vi "Parameter.vi"(9 "In":string, 10 "VIId":string, 11 "VariablesRef":T3) -> ()   [LabVIEW 2018, in "Array.lvlib"]
uses:
  Array.lvlib
  <userlib>/_OpenG.lib/dictionary/dictionary.llb/Dictionary Object RefNum__ogtk.ctl
  <userlib>/_OpenG.lib/dictionary/dictionary.llb/Dictionary Object RefNum - Enum__ogtk.ctl
  <vilib>/addons/_JKI.lib/Serialization/JSON/JKI JSON Serialization.lvlib
panel:
  in  "Tab Control":enum32{"Config", "控件"}(tab)
  in  "ArrayType":T1(tab)
  in  "索引_ArrayIndex":u32 caption="索引"
  in  "第一个元素_BuildArray":string(combo) caption="第一个元素"
  in  "第二个元素_BuildArray":string(combo) caption="第二个元素"
  in  "索引_InsertIntoArray":u32 caption="索引"
  in  "子数组_InsertIntoArray":string(combo) caption="子数组"
  in  "索引_DeleteFromArray":u32 caption="索引"
  in  "删除长度_DeleteFromArray":u32 caption="删除长度"
  in  "尺寸_InitializeArray":u32 caption="尺寸"
  in  "元素_InitializeArray":string(combo) caption="元素"
  in  "长度_ArraySubset":u32 caption="长度"
  in  "索引_ArraySubset":u32 caption="索引"
  in  "元素_SearchArray":string(combo) caption="元素"
  in  "起始索引_SearchArray":u32 caption="起始索引"
  in  "子数组_ReplaceArraySubset":string(combo) caption="子数组"
  in  "索引_ReplaceArraySubset":u32 caption="索引"
  in  "忽略NaN_ArrayAverage":bool
  in  "分隔符_ArrayToString":string(combo) caption="分隔符"
  in  "数组变量(ArrayVar)":u16(ring) items=["", "SN", "FileName", "ProductName", "TestLine", "TestStation"]
  in  "方法(Method)":T2(ring)
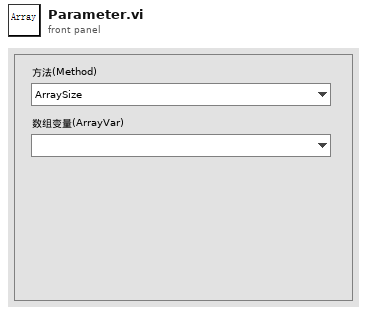
[diagram p1: front panel]
types:
  T1 = enum32{"ArraySize", "ArrayIndex", "BuildArray", "InsertIntoArray", "DeleteFromArray", "InitializeArray", "ArraySubset", "ArrayMax", "ArrayMin", "SearchArray", "ReplaceArraySubset", "SortArray", "ReverseArray", "ArrayAverage", "RemoveDuplicatesFromArray", "ArrayToString"}
  T2 = enum16{"ArraySize", "IndexArray", "BuildArray", "InsertIntoArray", "DeleteFromArray", "InitializeArray", "ArraySubset", "ArrayMax", "ArrayMin", "SearchArray", "ReplaceArraySubset", "SortArray", "ReverseArray", "ArrayAverage", "RemoveDuplicatesFromArray", "ArrayToString"}
  T3 = typedef "Dictionary Object RefNum__ogtk.ctl" = refnum<k1>
  T4 = cluster{"ArraySize":cluster{"json":cluster{"Method":string, "ArrayVar":string}}, "IndexArray":cluster{"json":cluster{"Method":string, "ArrayVar":string, "Index":i32}}, "BuildArray":cluster{"json":cluster{"Method":string, "FirstElementVar":string, "SecondElementVar":string}}, "InsertIntoArray":cluster{"json":cluster{"Method":string, "ArrayVar":string, "Index":i32, "SubArrayVar":string}}, "DeleteFromArray":cluster{"json":cluster{"Method":string, "ArrayVar":string, "Index":i32, "Length":i32}}, "InitializeArray":cluster{"json":cluster{"Method":string, "ElementVar":string, "DimensionSize":i32}}, "ArraySubset":cluster{"json":cluster{"Method":string, "ArrayVar":string, "Index":i32, "Length":i32}}, "ArrayMax":cluster{"json":cluster{"Method":string, "ArrayVar":string}}, "ArrayMin":cluster{"json":cluster{"Method":string, "ArrayVar":string}}, "SearchArray":cluster{"json":cluster{"Method":string, "ArrayVar":string, "ElementVar":string, "StartIndex":i32}}, "ReplaceArraySubset":cluster{"json":cluster{"Method":string, "ArrayVar":string, "Index":i32, "SubArrayVar":string}}, "SortArray":cluster{"json":cluster{"Method":string, "ArrayVar":string}}, "ReverseArray":cluster{"json":cluster{"Method":string, "ArrayVar":string}}, "ArrayAverage":cluster{"json":cluster{"Method":string, "NumArrayVar":string, "IgnoreNaN":bool}}, "RemoveDuplicatesFromArray":cluster{"json":cluster{"Method":string, "ArrayVar":string}}, "ArrayToString":cluster{"json":cluster{"Method":string, "ArrayVar":string, "Delimiter":string}}}
  T5 = enum32{"Invalid", "Standard", "Closed", "Hidden", "Minimized", "Maximized"}
  T6 = enum32{"invalid app kind", "Development System", "Run Time System", "Student Edition", "Embedded LabVIEW", "Evaluation", "Custom"}
  T7 = cluster{"Core":cluster{"Current VI Reference":refnum<vi>, "Close Panel on Exit?":bool}, "Parameter":cluster{"VariableRef":T3}, "Synchronize":cluster{"EnqueueData":cluster{"Action":enum16{"Create", "Query", "Revert", "UpdateVariable", "Close"}, "Data":variant}, "Echo":cluster{"VIRef":refnum<vi>, "JsonOut":string, "Status":string}, "Communicate":cluster{"ID":string, "JsonIn":string, "VarRef":T3}, "Queue":refnum<queue>}, "ArrayClusters":cluster{"ArraySize":cluster{"json":cluster{"Method":string, "ArrayVar":string}}, "IndexArray":cluster{"json":cluster{"Method":string, "ArrayVar":string, "Index":i32}}, "BuildArray":cluster{"json":cluster{"Method":string, "FirstElementVar":string, "SecondElementVar":string}}, "InsertIntoArray":cluster{"json":cluster{"Method":string, "ArrayVar":string, "Index":i32, "SubArrayVar":string}}, "DeleteFromArray":cluster{"json":cluster{"Method":string, "ArrayVar":string, "Index":i32, "Length":i32}}, "InitializeArray":cluster{"json":cluster{"Method":string, "ElementVar":string, "DimensionSize":i32}}, "ArraySubset":cluster{"json":cluster{"Method":string, "ArrayVar":string, "Index":i32, "Length":i32}}, "ArrayMax":cluster{"json":cluster{"Method":string, "ArrayVar":string}}, "ArrayMin":cluster{"json":cluster{"Method":string, "ArrayVar":string}}, "SearchArray":cluster{"json":cluster{"Method":string, "ArrayVar":string, "ElementVar":string, "StartIndex":i32}}, "ReplaceArraySubset":cluster{"json":cluster{"Method":string, "ArrayVar":string, "Index":i32, "SubArrayVar":string}}, "SortArray":cluster{"json":cluster{"Method":string, "ArrayVar":string}}, "ReverseArray":cluster{"json":cluster{"Method":string, "ArrayVar":string}}, "ArrayAverage":cluster{"json":cluster{"Method":string, "NumArrayVar":string, "IgnoreNaN":bool}}, "RemoveDuplicatesFromArray":cluster{"json":cluster{"Method":string, "ArrayVar":string}}, "ArrayToString":cluster{"json":cluster{"Method":string, "ArrayVar":string, "Delimiter":string}}}}
  T8 = cluster{"EnqueueData":cluster{"Action":enum16{"Create", "Query", "Revert", "UpdateVariable", "Close"}, "Data":variant}, "Echo":cluster{"VIRef":refnum<vi>, "JsonOut":string, "Status":string}, "Communicate":cluster{"ID":string, "JsonIn":string, "VarRef":T3}, "Queue":refnum<queue>}
  T9 = cluster{"Current VI Reference":refnum<vi>, "Close Panel on Exit?":bool}
  T10 = cluster{"json":cluster{"Method":string, "ArrayVar":string}}
  T11 = cluster{"json":cluster{"Method":string, "ArrayVar":string, "Index":i32}}
  T12 = cluster{"json":cluster{"Method":string, "FirstElementVar":string, "SecondElementVar":string}}
  T13 = cluster{"json":cluster{"Method":string, "ArrayVar":string, "Index":i32, "SubArrayVar":string}}
  T14 = cluster{"json":cluster{"Method":string, "ArrayVar":string, "Index":i32, "Length":i32}}
  T15 = cluster{"json":cluster{"Method":string, "ElementVar":string, "DimensionSize":i32}}
  T16 = cluster{"json":cluster{"Method":string, "ArrayVar":string, "ElementVar":string, "StartIndex":i32}}
  T17 = cluster{"json":cluster{"Method":string, "NumArrayVar":string, "IgnoreNaN":bool}}
  T18 = cluster{"json":cluster{"Method":string, "ArrayVar":string, "Delimiter":string}}
  T19 = cluster{"Action":enum16{"Create", "Query", "Revert", "UpdateVariable", "Close"}, "Data":variant}
  T20 = cluster{"ID":string, "JsonIn":string, "VarRef":T3}
  T21 = enum16{"Create", "Query", "Revert", "UpdateVariable", "Close"}
  T22 = cluster{"VIRef":refnum<vi>, "JsonOut":string, "Status":string}
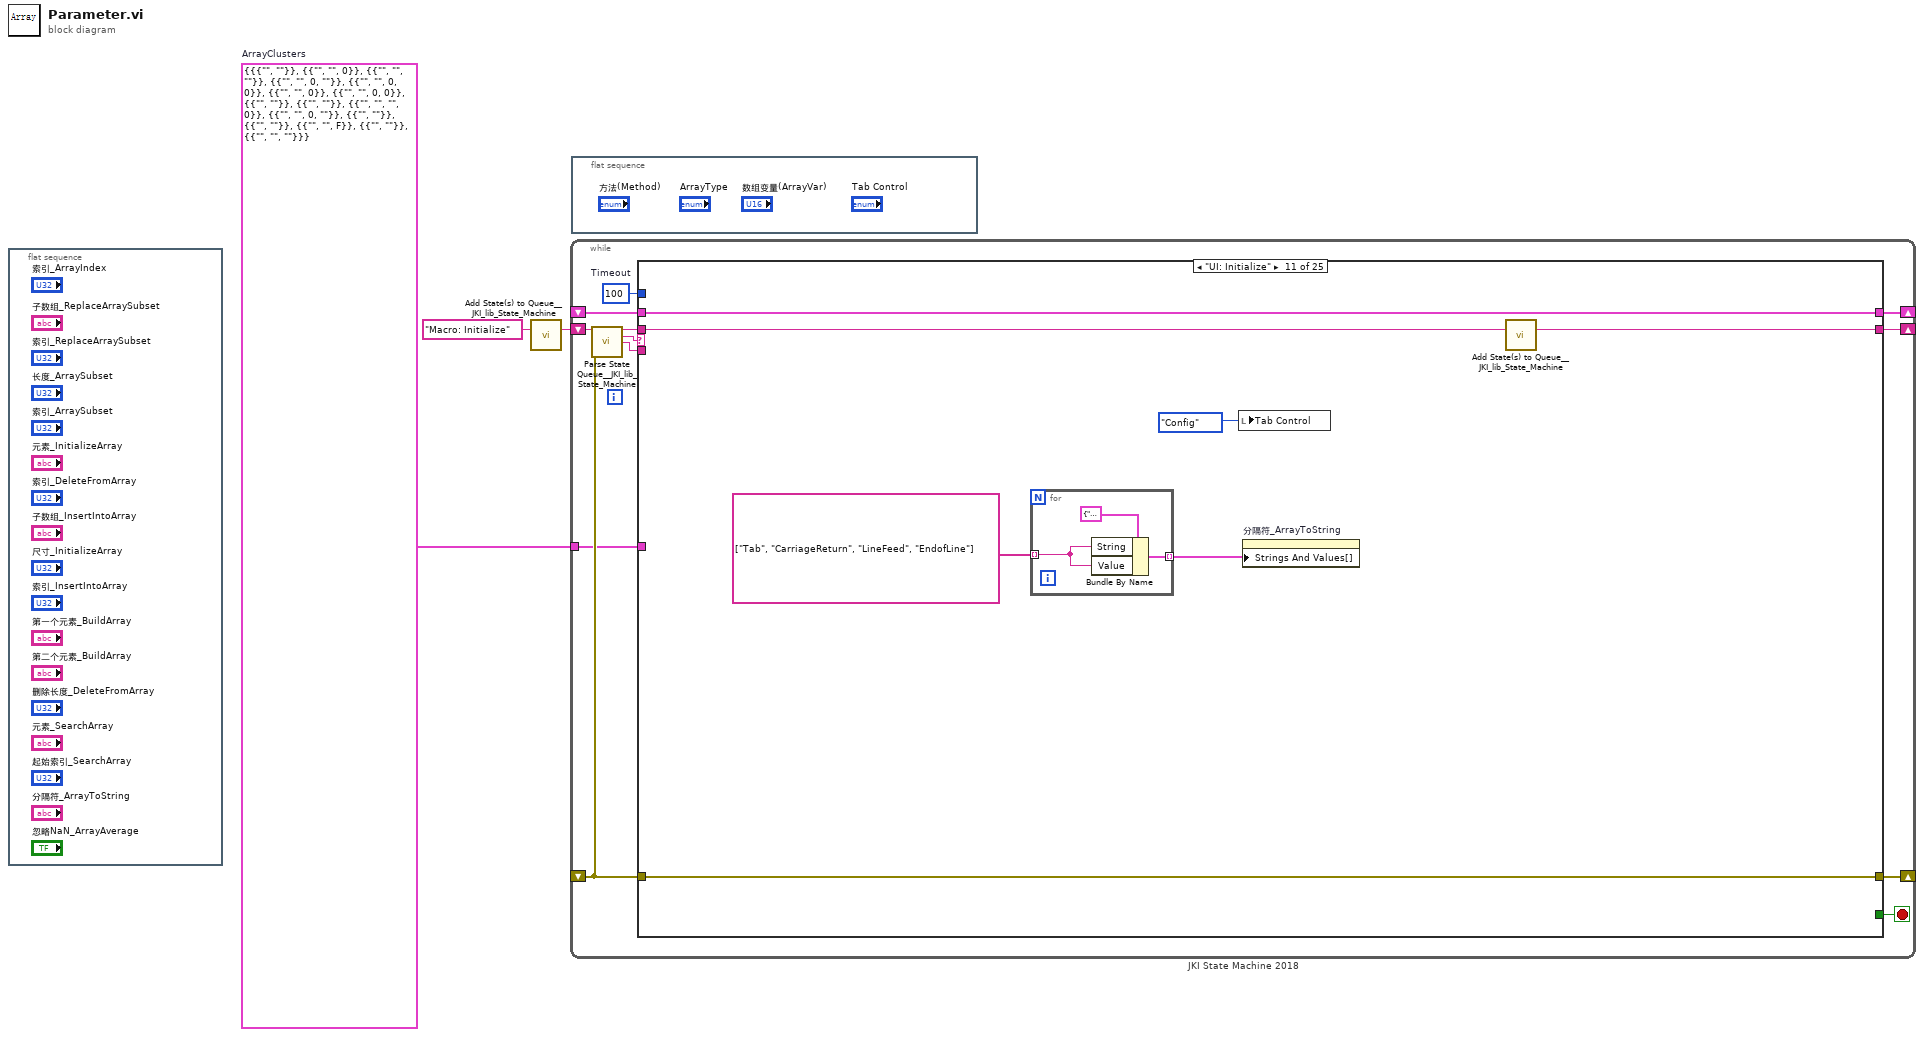
[diagram p0: block diagram]
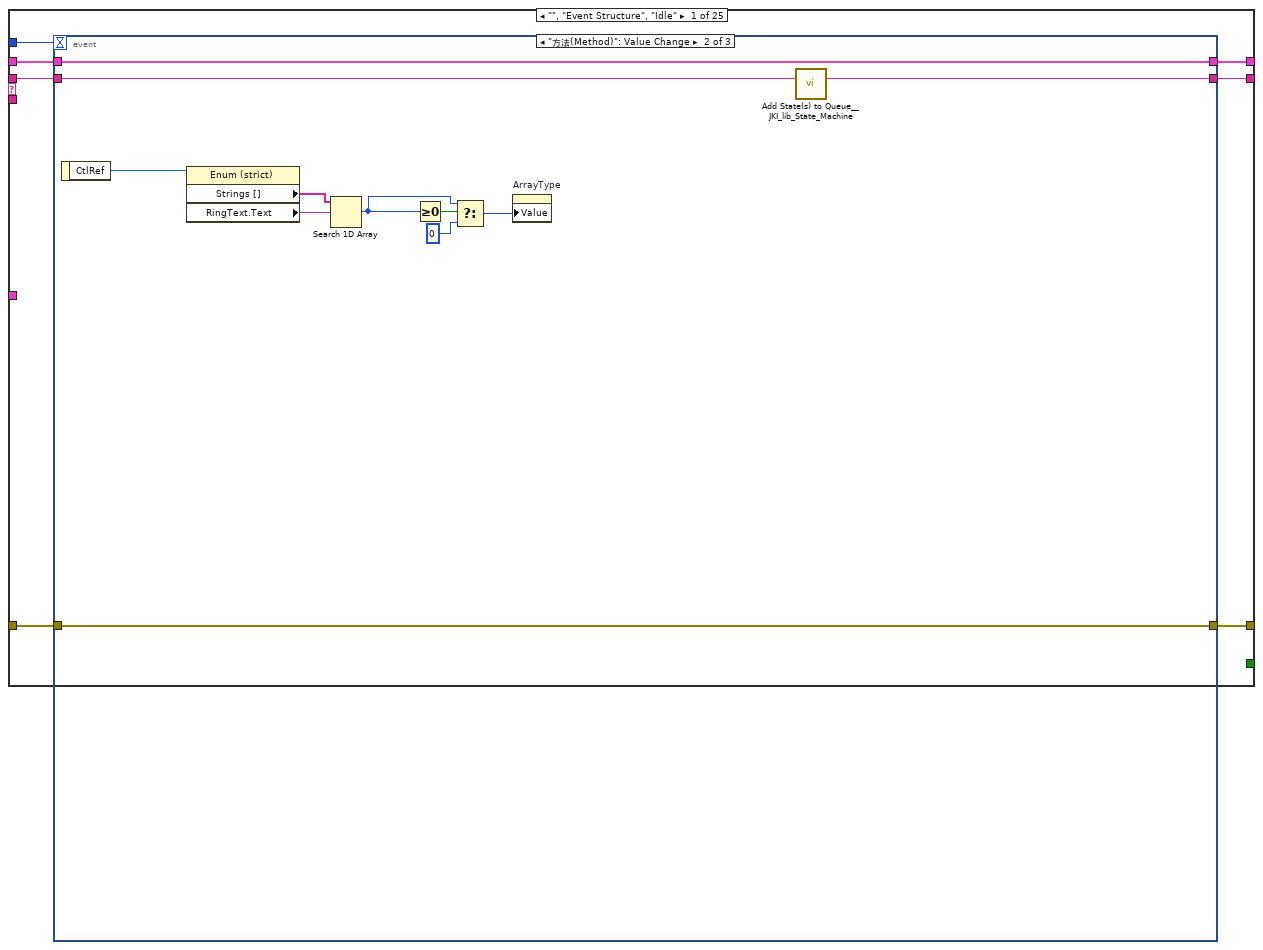
[diagram p2: hidden frame]
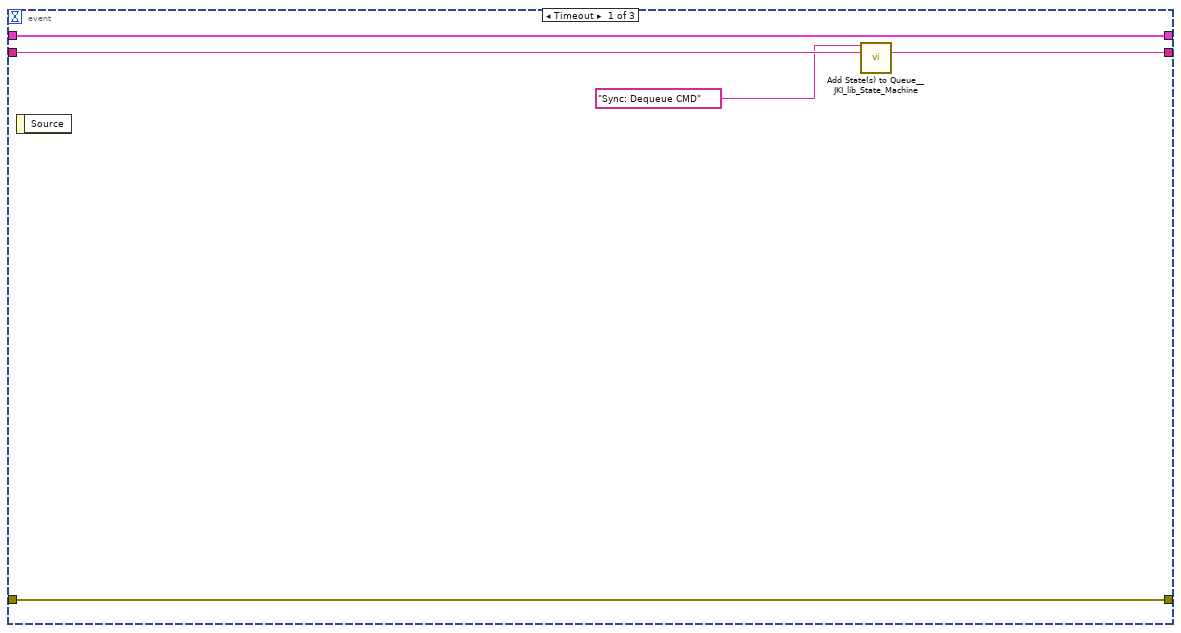
[diagram p3: hidden frame]
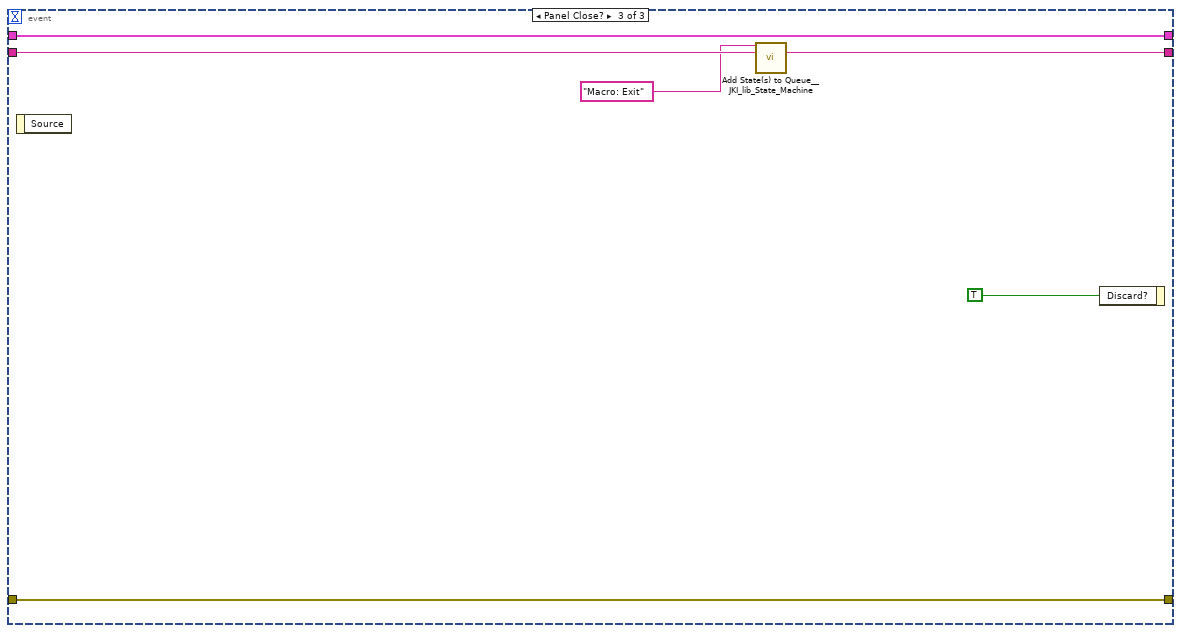
[diagram p4: hidden frame]
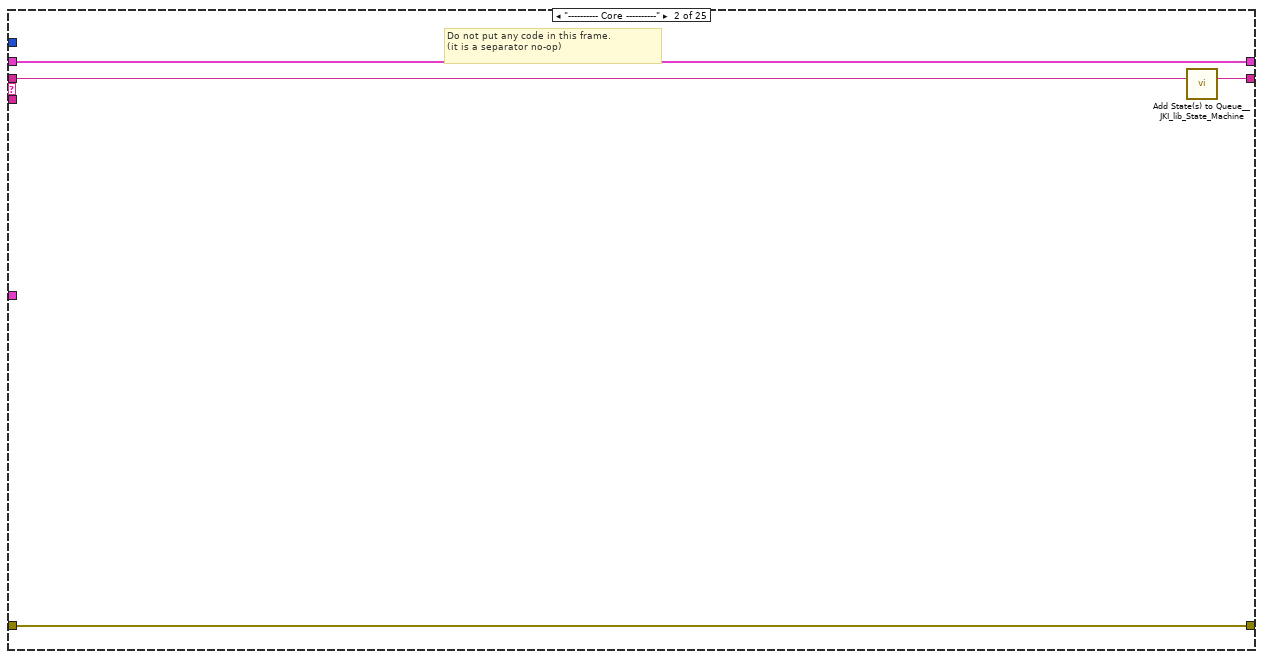
[diagram p5: hidden frame]
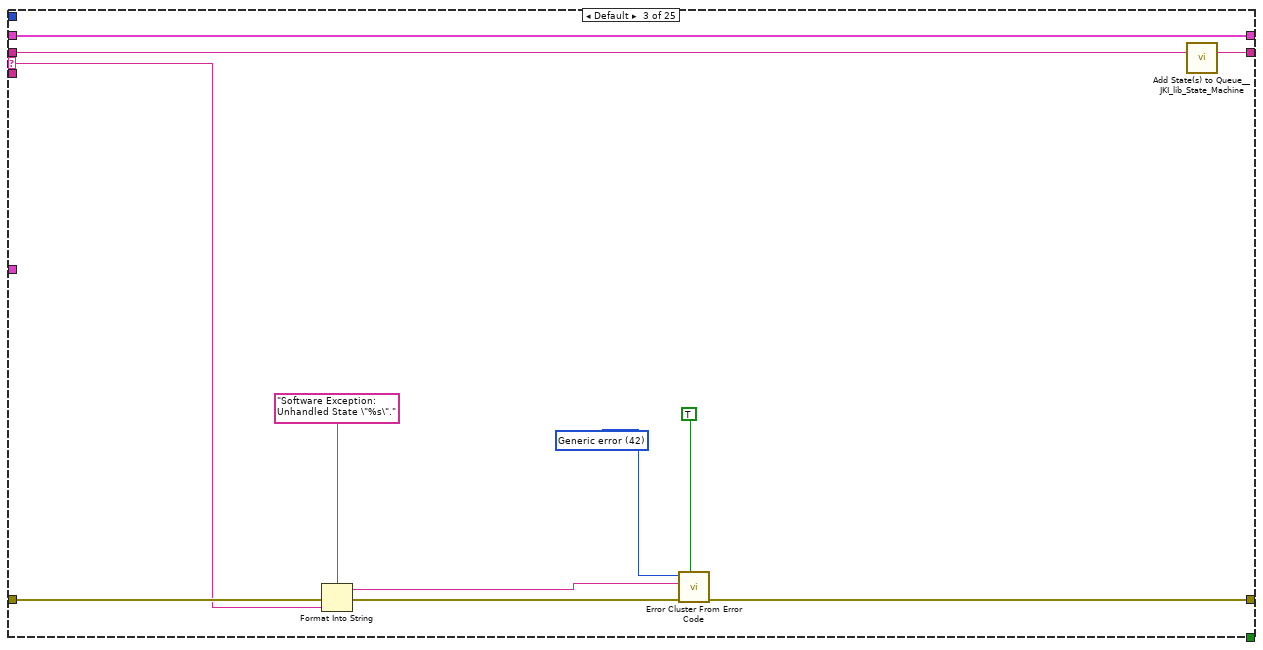
[diagram p6: hidden frame]
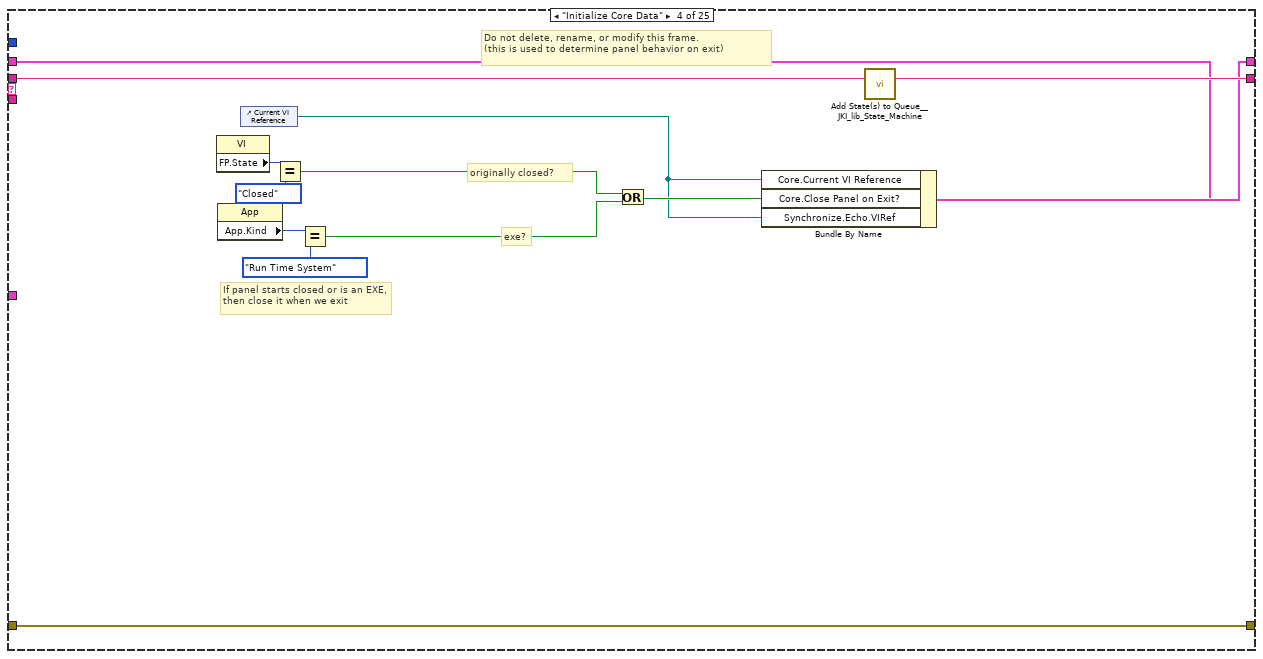
[diagram p7: hidden frame]
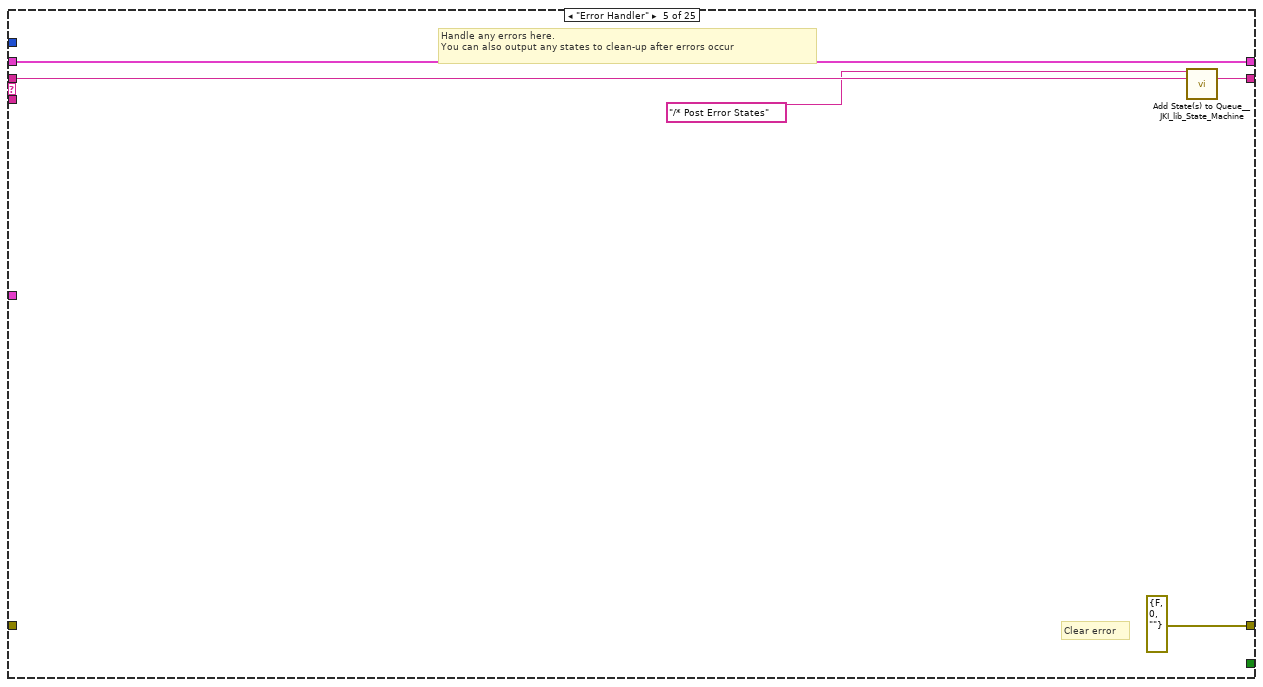
[diagram p8: hidden frame]
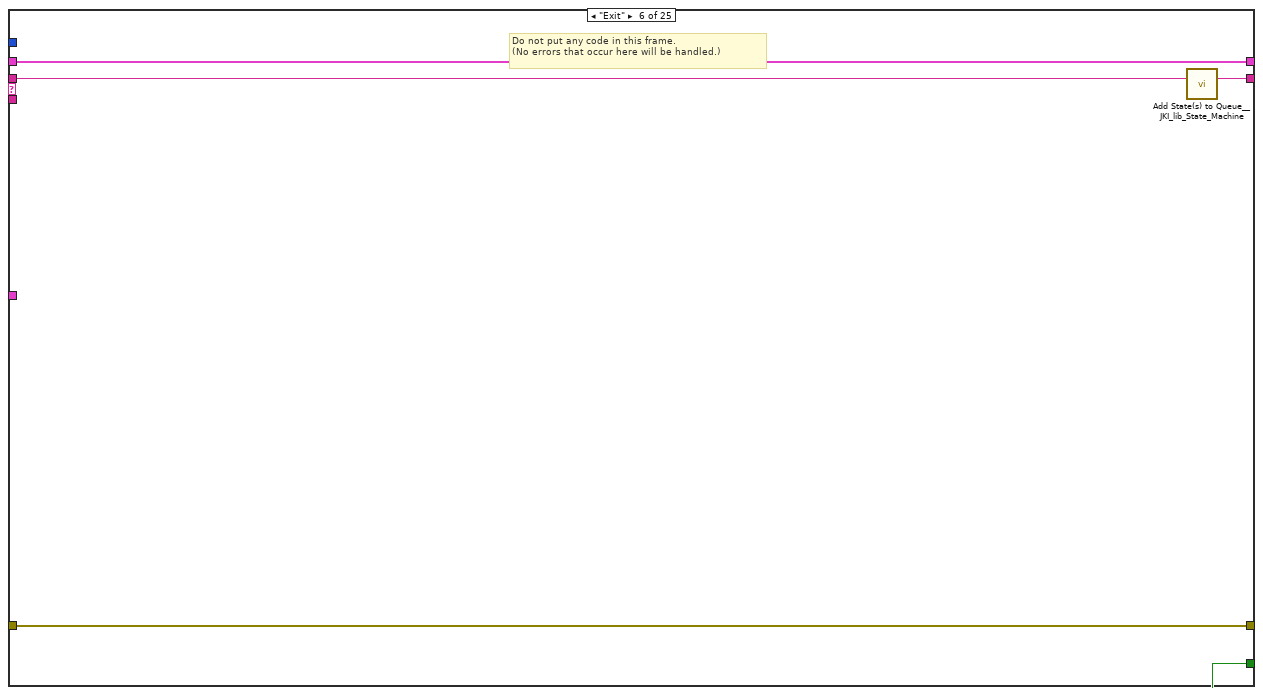
[diagram p9: hidden frame]
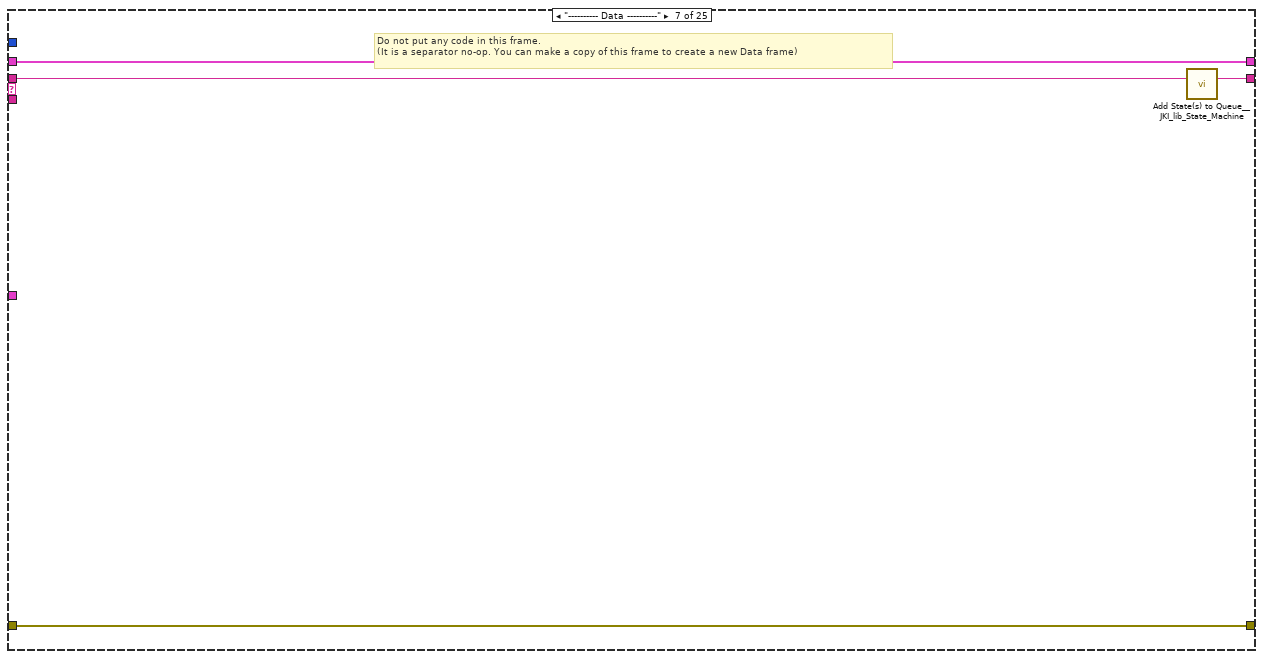
[diagram p10: hidden frame]
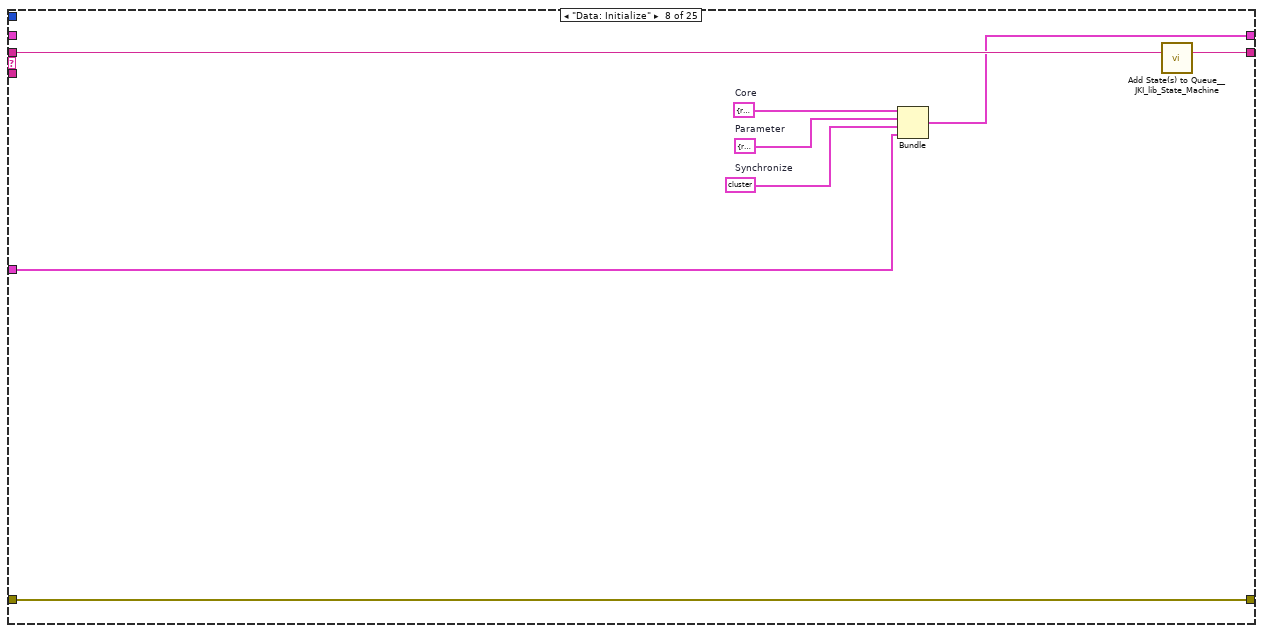
[diagram p11: hidden frame]
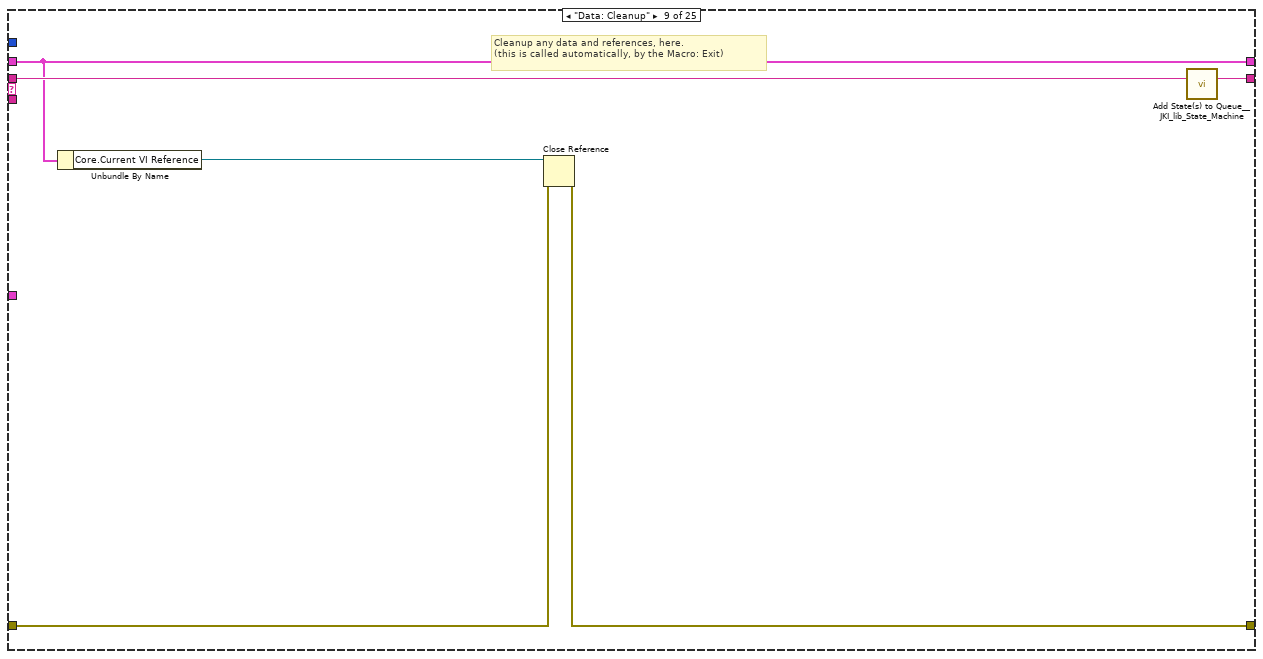
[diagram p12: hidden frame]
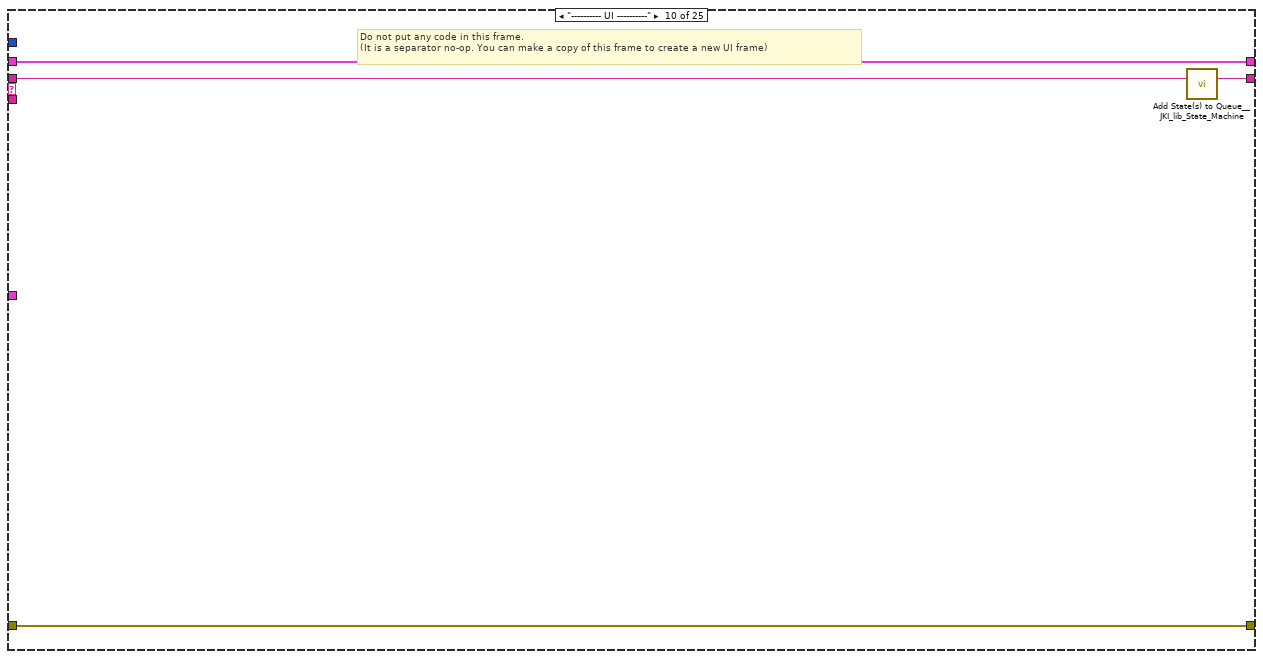
[diagram p13: hidden frame]
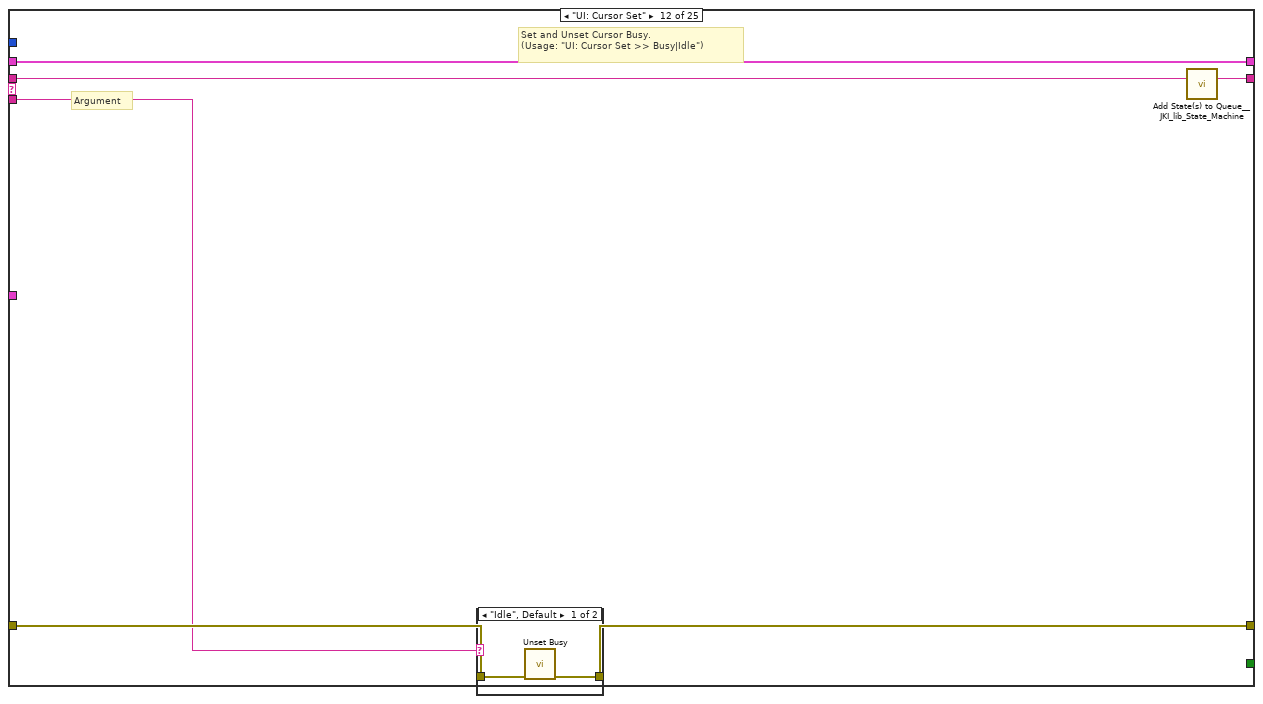
[diagram p14: hidden frame]
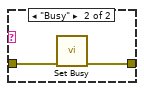
[diagram p15: hidden frame]
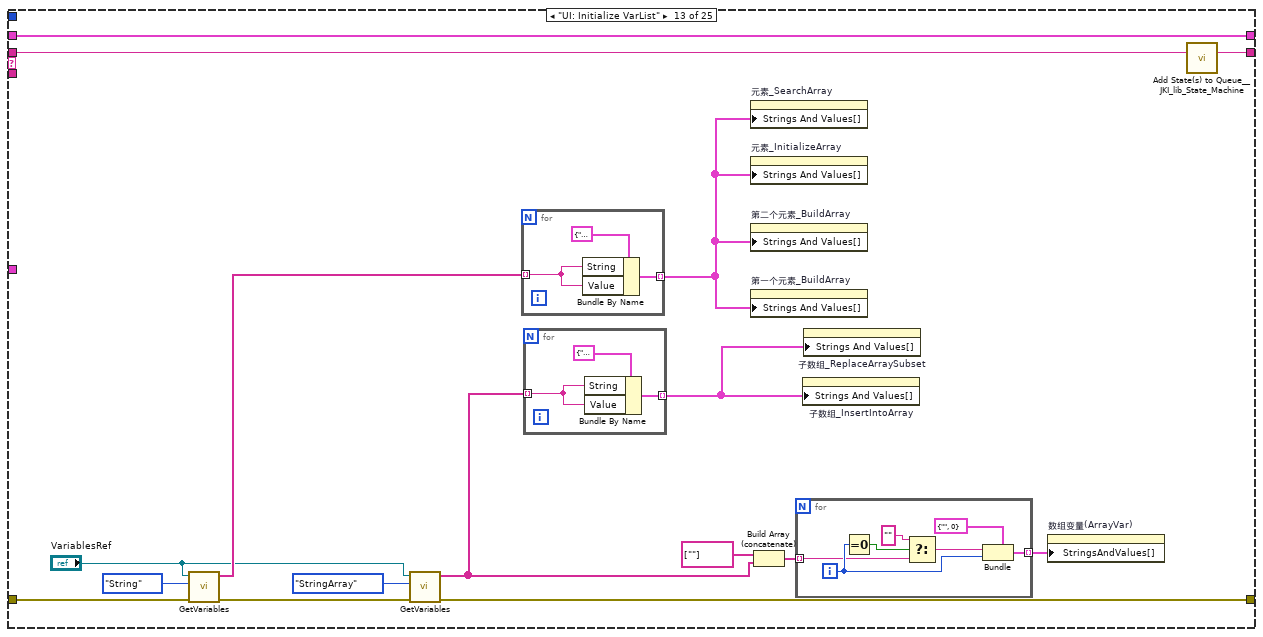
[diagram p16: hidden frame]
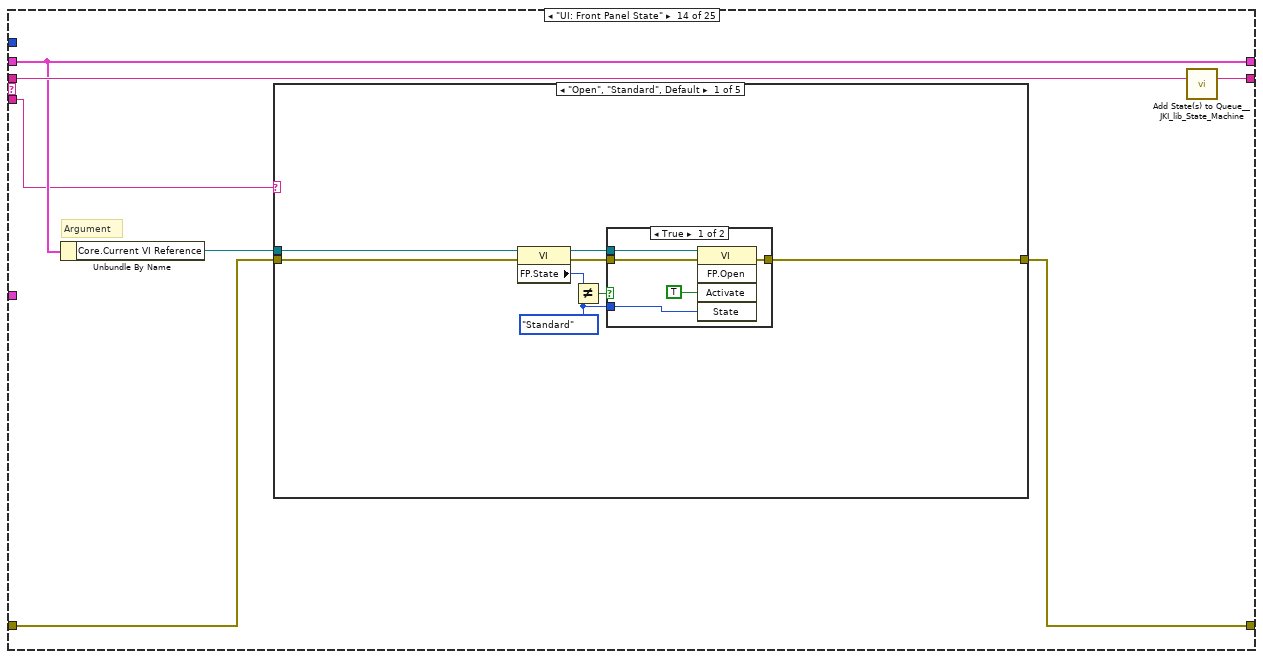
[diagram p17: hidden frame]
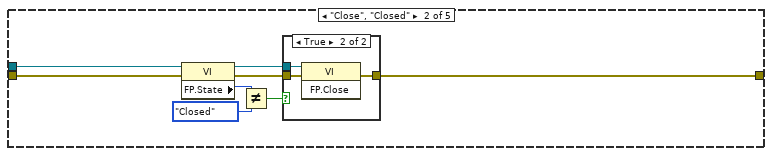
[diagram p19: hidden frame]
diagram:
  w1 = T4 {"ArraySize"={"json"={"Method"="", "ArrayVar"=""}}, "IndexArray"={"json"={"Method"="", "ArrayVar"="", "Index"=0}}, "BuildArray"={"json"={"Method"="", "FirstElementVar"="", "SecondElementVar"=""}}, "InsertIntoArray"={"json"={"Method"="", "ArrayVar"="", "Index"=0, "SubArrayVar"=""}}, "DeleteFromArray"={"json"={"Method"="", "ArrayVar"="", "Index"=0, "Length"=0}}, "InitializeArray"={"json"={"Method"="", "ElementVar"="", "DimensionSize"=0}}, "ArraySubset"={"json"={"Method"="", "ArrayVar"="", "Index"=0, "Length"=0}}, "ArrayMax"={"json"={"Method"="", "ArrayVar"=""}}, "ArrayMin"={"json"={"Method"="", "ArrayVar"=""}}, "SearchArray"={"json"={"Method"="", "ArrayVar"="", "ElementVar"="", "StartIndex"=0}}, "ReplaceArraySubset"={"json"={"Method"="", "ArrayVar"="", "Index"=0, "SubArrayVar"=""}}, "SortArray"={"json"={"Method"="", "ArrayVar"=""}}, "ReverseArray"={"json"={"Method"="", "ArrayVar"=""}}, "ArrayAverage"={"json"={"Method"="", "NumArrayVar"="", "IgnoreNaN"=FALSE}}, "RemoveDuplicatesFromArray"={"json"={"Method"="", "ArrayVar"=""}}, "ArrayToString"={"json"={"Method"="", "ArrayVar"="", "Delimiter"=""}}}  # ArrayClusters
  n1 = flat-sequence {
    frame #0 {
    }
  }
  n2 = call <vilib>:"Add State(s) to Queue__JKI_lib_State_Machine.vi"("State(s) in (\"\")"="Macro: Initialize") -> ("States Out"=w3:string)  [unwired: 14 in]
  n3 = while "JKI State Machine 2018" {
    shift-right: [w8] -> _
    shift-left: _ -> [w7]
    shift-right: [w11] -> _
    shift-left: _ -> [w5]
    shift-right: [w10] -> _
    shift-left: w3 -> [w12]
    tunnel: w1 -> [w4]
    stop <- w9 stop-if-true
    w6 = 100  # Timeout
    n4 = call <vilib>:"Parse State Queue__JKI_lib_State_Machine.vi"("State Queue"=w12, "Error In (no error)"=w5) -> ("Remaining States"=w14:string, "Current State"=w15:string, "Arguments"=w13:string)  [unwired: 11 in]
    n5 = case shown="\"UI: Initialize\"" w15 {
      selector: w15 -> [_ _ w49 _ _ _ _ _ _ _ _ _ _ _ _ _ _ _ _ _ _ _ _ _ _]
      tunnel: w14 -> [w22 w48 w53 w72 w77 w82 w86 w94 w100 w104 w111 w120 w140 w160 w229 w234 w244 w248 w256 w527 w691 w700 w715 w759 w774]
      tunnel: w13 -> [_ _ _ _ _ _ _ _ _ _ _ w115 _ w154 _ _ _ _ _ _ _ _ _ _ _]
      tunnel: w7 -> [w20 w45 w51 w65 w74 w80 w83 _ w95 w101 w108 w118 w138 w156 w226 w231 w241 w245 w251 w524 w688 w693 w713 w756 w763]
      tunnel: [w19 w46 w55 w69 errorcluster {"status"=FALSE, "code"=0, "source"=""} ("error out") w79 w84 w92 w96 w102 w107 w116 w137 w157 w227 w232 w242 w246 w252 w523 w689 w697 w702 w754 w761] -> w11
      tunnel: w5 -> [w18 w46 w54 w69 _ w79 w84 w92 w97 w102 w107 w117 w131 w158 w227 w232 w242 w246 w253 w522 w689 w698 w711 w755 w762]
      tunnel: [w21 w47 w52 w71 w76 w81 w85 w93 w99 w103 w110 w119 w139 w159 w228 w233 w243 w247 w255 w526 w690 w699 w714 w758 w773] -> w10
      tunnel: [_ _ _ _ _ TRUE _ _ _ _ _ _ _ _ _ _ _ _ _ _ _ _ _ _ _] -> w9
      tunnel: [w17 w45 w51 w70 w74 w80 w83 w89 w95 w101 w108 w118 w138 w156 w226 w231 w241 w245 w251 w525 w688 w695 w704 w756 w763] -> w8
      tunnel: w6 -> [w16 _ _ _ _ _ _ _ _ _ _ _ _ _ _ _ _ _ _ _ _ _ _ _ _]
      tunnel: w4 -> [_ _ _ _ _ _ _ w87 _ _ _ _ _ _ _ _ _ _ _ _ _ _ _ _ _]
      frame "", "Event Structure", "Idle" {
        n6 = event shown="[1] \"方法(Method)\": Value Change" {
          selector: _ -> [_ _ _]
          dyn-events: _ -> [_ _ _]
          timeout: w16 -> [_ _ _]
          tunnel: w22 -> [w27 w38 w44]
          tunnel: [w26 w37 w43] -> w21
          tunnel: w20 -> [w24 w35 w41]
          tunnel: [w25 w36 w42] -> w19
          tunnel: w18 -> [w25 w36 w42]
          tunnel: [w24 w35 w41] -> w17
          event Timeout {
            n7 = event-data() -> ()  [unwired: 1 in, 1 out]
            n8 = call <vilib>:"Add State(s) to Queue__JKI_lib_State_Machine.vi"("State(s) in Front (\"\")"="Sync: Dequeue CMD" ("State(s) in Front (\"\")"), "State(s) in (\"\")"=w27) -> ("States Out"=w26:string)  [unwired: 13 in]
          }
          event "方法(Method)": Value Change {
            n9 = event-data() -> ("CtlRef"=w31:refnum<vi>)  [unwired: 1 in]
            n10 = property class="Enum (strict)"(reference=w31) -> ("Strings []"=w30:string[], "RingText.Text"=w29:string)  [unwired: 1 in, 2 out]
            n11 = Search 1D Array(1D array=w30, element=w29) -> (index of element=w33:i32)  [unwired: 1 in]
            n12 = Greater Or Equal To 0?(x=w33) -> (x >= 0?=w34:bool)
            n13 = Select(t=w33, s=w34, f=0) -> (s? t:f=w28:i32)
            n14 = property on="ArrayType" class="TabCtl (strict)"("Value"=w28) -> ()  [unwired: 2 in, 2 out]
            n15 = call <vilib>:"Add State(s) to Queue__JKI_lib_State_Machine.vi"("State(s) in (\"\")"=w38) -> ("States Out"=w37:string)  [unwired: 14 in]
          }
          event Panel Close? {
            n16 = event-data() -> ()  [unwired: 1 in, 1 out]
            n17 = call <vilib>:"Add State(s) to Queue__JKI_lib_State_Machine.vi"("State(s) in Front (\"\")"="Macro: Exit", "State(s) in (\"\")"=w44) -> ("States Out"=w43:string)  [unwired: 13 in]
            n18 = event-data("Discard?"=TRUE) -> ()  [unwired: 1 in, 1 out]
          }
        }
      }
      frame "---------- Core ----------" {
        # "Do not put any code in this frame.\n(it is a separator no-op)"
        n19 = call <vilib>:"Add State(s) to Queue__JKI_lib_State_Machine.vi"("State(s) in (\"\")"=w48) -> ("States Out"=w47:string)  [unwired: 14 in]
      }
      frame Default {
        w58 = 42 items=["No error", "Argument error", "Memory is full", "Out of zone", "End of file", "File already open", "Generic file I/O error", "File not found", "File permission error", "Disk is full", "Duplicate path", "Too many files open", "System feature not enabled", "Resource file not found", "Cannot add resource", "Resource not found", "Image not found", "Image memory error", "Pen does not exist", "Config type invalid", "Config token not found", "Config parse error", "Config memory error", "Bad external code format", "Bad external code offset", "External code not present", "Null window", "Destroy window error", "Null menu", "Print aborted", "Bad print record", "Print driver error", "Windows error during printing", "Memory error during printing", "Print dialog error", "Generic print error", "Invalid device refnum", "Device not found", "Device parameter error", "Device unit error", "Cannot open device", "Device call aborted", "Generic error", "Cancelled by user", "Object ID too low", "Object ID too high", "Object not in heap", "Unknown heap", "Unknown object (invalid DefProc)", "Unknown object (DefProc not in table)", "Message out of range", "Invalid (null) method", "Unknown message", "Manager call not supported", "Bad address", "Network operation in progress", "Network operation timed out", "Connection is busy", "Network attribute not supported", "Network error", "Address in use", "System out of memory", "Connection aborted", "Connection refused", "Not connected", "Already connected", "Connection closed", "Initialization error (interapplication manager)", "Bad occurrence", "Wait on unbound occurrence handler", "Occurrence queue overflow", "Datalog type conflict", "Unused", "Unrecognized type (interapplication manager)", "Memory corrupt", "Failed to make temporary DLL", "Old CIN version", "Drag socket not found", "Failed to load drop-object", "Failed to register OLE object", "Failed to release OLE object", "Format specifier type mismatch", "Unknown format specifier", "Too few format specifiers", "Too many format specifiers", "Scan failed", "Newer CIN version", "Error converting to variant", "Runtime menu error", "Password tampered", "Variant attribute not found", "Incompatible variant data type", "Event data is not available", "Event Store is not present", "Occurrence is not found", "Event Queue is not created", "Event info is not available", "Refnum passed is NULL", "Error retrieving Class GUID", "Error retrieving CoClass GUID", "Error retrieving TypeLib GUID.", "Bad built application magic bytes.", "Specific driver is different from the specific driver associated with the Logical Name.", "There is no session opened to the class driver.", "Max Error", "MAX - Error with config objects", "MAX - Error loading configuration", "MAX - Group not supported"]
        n20 = Format Into String(format string="Software Exception: Unhandled State \"%s\"." ("message"), error in=w54, w49) -> (resulting string=w57:string, error out=w56:errorcluster)  [unwired: 1 in]
        n21 = call <vilib>:"Error Cluster From Error Code.vi"("show call chain? (False)"=TRUE, "error in (no error)"=w56, "error message (\"\")"=w57, "error code (0)"=w58) -> ("error out"=w55:errorcluster)  [unwired: 5 in]
        n22 = call <vilib>:"Add State(s) to Queue__JKI_lib_State_Machine.vi"("State(s) in (\"\")"=w53) -> ("States Out"=w52:string)  [unwired: 14 in]
      }
      frame "Initialize Core Data" {
        # "Do not delete, rename, or modify this frame.\n(this is used to determine panel behavior on exit)"
        # "originally closed?"
        # "exe?"
        # "If panel starts closed or is an EXE, then close it when we exit"
        n23 = property class="VI"() -> ("FP.State"=w63:T5)  [unwired: 2 in, 2 out]
        n24 = property class="App"() -> ("App.Kind"=w68:T6)  [unwired: 2 in, 2 out]
        n25 = control-ref of="Current VI Reference"() -> (w60:refnum<vi>)
        n26 = Equal?(x=w63, y=T5."Closed" ("Front Panel Window:State")) -> (x = y?=w61:bool)
        n27 = Equal?(x=w68, y=T6."Run Time System" ("Application:Kind")) -> (x = y?=w66:bool)
        n28 = Or(x=w61, y=w66) -> (x .or. y?=w64:bool)
        n29 = Bundle By Name(cluster=w65, "Core.Current VI Reference"=w60, "Core.Close Panel on Exit?"=w64, "Synchronize.Echo.VIRef"=w60) -> (w70:T7)
        n30 = call <vilib>:"Add State(s) to Queue__JKI_lib_State_Machine.vi"("State(s) in (\"\")"=w72) -> ("States Out"=w71:string)  [unwired: 14 in]
      }
      frame "Error Handler" {
        # "Handle any errors here.\nYou can also output any states to clean-up after errors occur"
        # "Clear error"
        n31 = call <vilib>:"Add State(s) to Queue__JKI_lib_State_Machine.vi"("State(s) in Front (\"\")"="/* Post Error States", "State(s) in (\"\")"=w77) -> ("States Out"=w76:string)  [unwired: 13 in]
      }
      frame "Exit" {
        # "Do not put any code in this frame.\n(No errors that occur here will be handled.)"
        n32 = call <vilib>:"Add State(s) to Queue__JKI_lib_State_Machine.vi"("State(s) in (\"\")"=w82) -> ("States Out"=w81:string)  [unwired: 14 in]
      }
      frame "---------- Data ----------" {
        # "Do not put any code in this frame.\n(It is a separator no-op. You can make a copy of this frame to create a new Data frame)"
        n33 = call <vilib>:"Add State(s) to Queue__JKI_lib_State_Machine.vi"("State(s) in (\"\")"=w86) -> ("States Out"=w85:string)  [unwired: 14 in]
      }
      frame "Data: Initialize" {
        w88 = cluster{"VariableRef":T3} {"VariableRef"=refnum}  # Parameter
        w90 = T8 {"EnqueueData"={"Action"=enum."Create", "Data"=variant}, "Echo"={"VIRef"=refnum, "JsonOut"="", "Status"=""}, "Communicate"={"ID"="", "JsonIn"="", "VarRef"=refnum}, "Queue"=refnum}  # Synchronize
        w91 = T9 {"Current VI Reference"=refnum, "Close Panel on Exit?"=FALSE}  # Core
        n34 = Bundle("Core"=w91, "Parameter"=w88, "Synchronize"=w90, "ArrayClusters"=w87) -> (w89:T7)  [unwired: 1 in]
        n35 = call <vilib>:"Add State(s) to Queue__JKI_lib_State_Machine.vi"("State(s) in (\"\")"=w94) -> ("States Out"=w93:string)  [unwired: 14 in]
      }
      frame "Data: Cleanup" {
        # "Cleanup any data and references, here.\n(this is called automatically, by the Macro: Exit)"
        n36 = Unbundle By Name(w95) -> ("Core.Current VI Reference"=w98:refnum<vi>)
        n37 = Close Reference(reference=w98, error in (no error)=w97) -> (error out=w96:errorcluster)
        n38 = call <vilib>:"Add State(s) to Queue__JKI_lib_State_Machine.vi"("State(s) in (\"\")"=w100) -> ("States Out"=w99:string)  [unwired: 14 in]
      }
      frame "---------- UI ----------" {
        # "Do not put any code in this frame.\n(It is a separator no-op. You can make a copy of this frame to create a new UI frame)"
        n39 = call <vilib>:"Add State(s) to Queue__JKI_lib_State_Machine.vi"("State(s) in (\"\")"=w104) -> ("States Out"=w103:string)  [unwired: 14 in]
      }
      frame "UI: Initialize" {
        n40 = for {
          tunnel: string[] ["Tab", "CarriageReturn", "LineFeed", "EndofLine"] -> [w112] mode=indexing
          tunnel: [w113] -> w106 mode=indexing
          n41 = Bundle By Name(cluster=cluster{"String":string, "Value":string} {"String"="", "Value"=""}, "String"=w112, "Value"=w112) -> (w113:cluster{"String":string, "Value":string})
        }
        n42 = local write "Tab Control"(enum32{"Config", "控件"}."Config" ("Tab Control")) -> ()
        n43 = property on="分隔符_ArrayToString" class="CmbBox"("Strings And Values[]"=w106) -> ()  [unwired: 2 in, 2 out]
        n44 = call <vilib>:"Add State(s) to Queue__JKI_lib_State_Machine.vi"("State(s) in (\"\")"=w111) -> ("States Out"=w110:string)  [unwired: 14 in]
      }
      frame "UI: Cursor Set" {
        # "Argument"
        # "Set and Unset Cursor Busy.\n(Usage: \"UI: Cursor Set >> Busy|Idle\")"
        n45 = case shown="\"Idle\", Default" w115 {
          tunnel: w117 -> [w122 w124]
          tunnel: [w121 w123] -> w116
          frame "Idle", Default {
            n46 = call <vilib>:"Unset Busy.vi"("error in (no error)"=w122) -> ("error out"=w121:errorcluster)  [unwired: 10 in]
          }
          frame "Busy" {
            n47 = call <vilib>:"Set Busy.vi"("error in (no error)"=w124) -> ("error out"=w123:errorcluster)  [unwired: 9 in, 1 out]
          }
        }
        n48 = call <vilib>:"Add State(s) to Queue__JKI_lib_State_Machine.vi"("State(s) in (\"\")"=w120) -> ("States Out"=w119:string)  [unwired: 14 in]
      }
      frame "UI: Initialize VarList" {
        n49 = call "GetVariables.vi"("error in (no error)"=w131, "VariableType"=enum16{"String", "StringArray"}."String", "DicRef"="VariablesRef") -> ("error out"=w130:errorcluster, "VariableArray"=w129:string[])  [unwired: 7 in]
        n50 = call "GetVariables.vi"("error in (no error)"=w130, "VariableType"=enum16{"String", "StringArray"}."StringArray", "DicRef"="VariablesRef") -> ("error out"=w137:errorcluster, "VariableArray"=w127:string[])  [unwired: 7 in]
        n51 = for {
          tunnel: w129 -> [w144] mode=indexing
          tunnel: [w145] -> w126 mode=indexing
          n52 = Bundle By Name(cluster=cluster{"String":string, "Value":string} {"String"="", "Value"=""}, "String"=w144, "Value"=w144) -> (w145:cluster{"String":string, "Value":string})
        }
        n53 = for {
          tunnel: w127 -> [w141] mode=indexing
          tunnel: [w142] -> w125 mode=indexing
          n54 = Bundle By Name(cluster=cluster{"String":string, "Value":string} {"String"="", "Value"=""}, "String"=w141, "Value"=w141) -> (w142:cluster{"String":string, "Value":string})
        }
        n55 = property on="元素_SearchArray" class="CmbBox"("Strings And Values[]"=w126) -> ()  [unwired: 2 in, 2 out]
        n56 = property on="元素_InitializeArray" class="CmbBox"("Strings And Values[]"=w126) -> ()  [unwired: 2 in, 2 out]
        n57 = property on="第二个元素_BuildArray" class="CmbBox"("Strings And Values[]"=w126) -> ()  [unwired: 2 in, 2 out]
        n58 = property on="第一个元素_BuildArray" class="CmbBox"("Strings And Values[]"=w126) -> ()  [unwired: 2 in, 2 out]
        n59 = Build Array (concatenate)(string[] [""] ("array"), w127) -> (w135:string[])
        n60 = for {
          tunnel: [w152] -> w133 mode=indexing
          tunnel: w135 -> [w147] mode=indexing
          i -> [w151]
          n61 = Equal To 0?(x=w151) -> (x = 0?=w150:bool)
          n62 = Select(t="", s=w150, f=w147) -> (s? t:f=w149:string)
          n63 = Bundle(cluster=cluster{"String":string, "Value":u16} {"String"="", "Value"=0}, "String"=w149, "Value"=w151) -> (w152:cluster{"String":string, "Value":u16})
        }
        n64 = property on="子数组_InsertIntoArray" class="CmbBox"("Strings And Values[]"=w125) -> ()  [unwired: 2 in, 2 out]
        n65 = property on="子数组_ReplaceArraySubset" class="CmbBox"("Strings And Values[]"=w125) -> ()  [unwired: 2 in, 2 out]
        n66 = property on="数组变量(ArrayVar)" class="Ring (strict)"("StringsAndValues[]"=w133) -> ()  [unwired: 2 in, 2 out]
        n67 = call <vilib>:"Add State(s) to Queue__JKI_lib_State_Machine.vi"("State(s) in (\"\")"=w140) -> ("States Out"=w139:string)  [unwired: 14 in]
      }
      frame "UI: Front Panel State" {
        # "Argument"
        n68 = Unbundle By Name(w156) -> ("Core.Current VI Reference"=w155:refnum<vi>)
        n69 = case shown="\"Open\", \"Standard\", Default" w154 {
          tunnel: w158 -> [w166 w181 w192 w205 w218]
          tunnel: [w168 w182 w194 w207 w220] -> w157
          tunnel: w155 -> [w167 w179 w193 w206 w219]
          frame "Open", "Standard", Default {
            w161 = T5."Standard" ("State")
            n70 = property class="VI"(reference=w167, error in=w166) -> (reference out=w164:refnum<vi>, error out=w165:errorcluster, "FP.State"=w163:T5)
            n71 = Not Equal?(x=w163, y=w161) -> (x != y?=w162:bool)
            n72 = case shown="True" w162 {
              tunnel: [w172 w174] -> w168
              tunnel: w165 -> [w171 w174]
              tunnel: w164 -> [w170 _]
              tunnel: w161 -> [w169 _]
              frame True {
                n73 = invoke class="VI" method="FP.Open"(reference=w170, error in=w171, "Activate"=TRUE, "State"=w169) -> (error out=w172:errorcluster)  [unwired: 1 in, 4 out]
              }
              frame False {
              }
            }
          }
          frame "Close", "Closed" {
            n74 = property class="VI"(reference=w179, error in=w181) -> (reference out=w178:refnum<vi>, error out=w180:errorcluster, "FP.State"=w176:T5)
            n75 = Not Equal?(x=w176, y=T5."Closed" ("Front Panel Window:State")) -> (x != y?=w175:bool)
            n76 = case shown="True" w175 {
              tunnel: [w183 w186] -> w182
              tunnel: w180 -> [w183 w185]
              tunnel: w178 -> [_ w184]
              frame False {
              }
              frame True {
                n77 = invoke class="VI" method="FP.Close"(reference=w184, error in=w185) -> (error out=w186:errorcluster)  [unwired: 1 in, 2 out]
              }
            }
          }
          frame "Hidden", "Hide" {
            w187 = T5."Hidden" ("State")
            n78 = property class="VI"(reference=w193, error in=w192) -> (reference out=w190:refnum<vi>, error out=w191:errorcluster, "FP.State"=w189:T5)
            n79 = Not Equal?(x=w189, y=w187) -> (x != y?=w188:bool)
            n80 = case shown="True" w188 {
              tunnel: [w198 w199] -> w194
              tunnel: w191 -> [w197 w199]
              tunnel: w190 -> [w196 _]
              tunnel: w187 -> [w195 _]
              frame True {
                n81 = invoke class="VI" method="FP.Open"(reference=w196, error in=w197, "State"=w195) -> (error out=w198:errorcluster)  [unwired: 2 in, 4 out]
              }
              frame False {
              }
            }
          }
          frame "Minimize", "Minimized" {
            w200 = T5."Minimized" ("State")
            n82 = property class="VI"(reference=w206, error in=w205) -> (reference out=w203:refnum<vi>, error out=w204:errorcluster, "FP.State"=w202:T5)
            n83 = Not Equal?(x=w202, y=w200) -> (x != y?=w201:bool)
            n84 = case shown="True" w201 {
              tunnel: [w211 w212] -> w207
              tunnel: w204 -> [w210 w212]
              tunnel: w203 -> [w209 _]
              tunnel: w200 -> [w208 _]
              frame True {
                n85 = invoke class="VI" method="FP.Open"(reference=w209, error in=w210, "State"=w208) -> (error out=w211:errorcluster)  [unwired: 2 in, 4 out]
              }
              frame False {
              }
            }
          }
          frame "Maximize", "Maximized" {
            w213 = T5."Maximized" ("State")
            n86 = property class="VI"(reference=w219, error in=w218) -> (reference out=w216:refnum<vi>, error out=w217:errorcluster, "FP.State"=w215:T5)
            n87 = Not Equal?(x=w215, y=w213) -> (x != y?=w214:bool)
            n88 = case shown="True" w214 {
              tunnel: [w224 w225] -> w220
              tunnel: w217 -> [w223 w225]
              tunnel: w216 -> [w222 _]
              tunnel: w213 -> [w221 _]
              frame True {
                n89 = invoke class="VI" method="FP.Open"(reference=w222, error in=w223, "State"=w221) -> (error out=w224:errorcluster)  [unwired: 2 in, 4 out]
              }
              frame False {
              }
            }
          }
        }
        n90 = call <vilib>:"Add State(s) to Queue__JKI_lib_State_Machine.vi"("State(s) in (\"\")"=w160) -> ("States Out"=w159:string)  [unwired: 14 in]
      }
      frame "---------- Macro ----------" {
        n91 = call <vilib>:"Add State(s) to Queue__JKI_lib_State_Machine.vi"("State(s) in (\"\")"=w229) -> ("States Out"=w228:string)  [unwired: 14 in]
      }
      frame "Macro: Initialize" {
        n92 = call <vilib>:"Add State(s) to Queue__JKI_lib_State_Machine.vi"("State(s) in Front (\"\")"="Data: Initialize\nInitialize Core Data\nUI: Initialize\nSync: Obtain CMD Queue\nSync: Dequeue CMD\nUI: Initialize VarList\nParameter: Parse Parameter", "State(s) in (\"\")"=w234) -> ("States Out"=w233:string)  [unwired: 13 in]
      }
      frame "Macro: Exit" {
        n93 = Unbundle By Name(w241) -> ("Core.Close Panel on Exit?"=w240:bool)
        n94 = Select(t="UI: Front Panel State >> Close", s=w240, f="") -> (s? t:f=w237:string)
        n95 = call <vilib>:"Add State(s) to Queue__JKI_lib_State_Machine.vi"("State(s) in (\"\")"=w237, "State(s) at Back (\"\")"="Sync: Release CMD Queue\nData: Cleanup\nExit") -> ("States Out"=w235:string)  [unwired: 13 in]
        n96 = call <vilib>:"Add State(s) to Queue__JKI_lib_State_Machine.vi"("State(s) in Front (\"\")"=w235, "State(s) in (\"\")"=w244) -> ("States Out"=w243:string)  [unwired: 13 in]
      }
      frame "---------- Parameter ----------" {
        # "Template Separator\n(You can make a copy of, or modify, this frame)"
        n97 = call <vilib>:"Add State(s) to Queue__JKI_lib_State_Machine.vi"("State(s) in (\"\")"=w248) -> ("States Out"=w247:string)  [unwired: 14 in]
      }
      frame "Parameter: Parse Parameter" {
        n98 = Unbundle By Name(w251) -> ("ArrayClusters"=w250:T4)
        n99 = Empty String/Path?(string/path="In") -> (empty?=w254:bool)
        n100 = case shown="False" w254 {
          tunnel: "In" -> [w265 _]
          tunnel: w253 -> [w270 w519]
          tunnel: [w269 w519] -> w252
          tunnel: w250 -> [w268 _]
          frame False {
            n101 = Match Pattern(string=w265, regular expression="\"Method\":\"") -> (after substring=w264:string)  [unwired: 1 in, 3 out]
            n102 = Match Pattern(string=w264, regular expression="\",") -> (before substring=w263:string)  [unwired: 1 in, 3 out]
            n103 = case shown="\"InsertIntoArray\"" w263 {
              tunnel: w265 -> [w283 w299 w311 w328 w345 w357 w374 w389 w404 w421 w438 w453 w468 w484 w499 w515 _]
              tunnel: w270 -> [w281 w297 w309 w326 w343 w355 w372 w387 w402 w419 w436 w451 w466 w482 w497 w513 w518]
              tunnel: [w280 w296 w308 w325 w342 w354 w371 w386 w401 w418 w435 w450 w465 w481 w496 w512 w518] -> w269
              tunnel: w268 -> [w272 w287 w306 w323 w340 w352 w369 w384 w399 w416 w433 w448 w463 w479 w494 w510 _]
              tunnel: [w273 w288 w307 w324 w341 w353 w370 w385 w400 w417 w434 w449 w464 w480 w495 w511 _] -> w258
              frame "ArraySize" {
                n104 = Unbundle By Name(w272) -> ("ArraySize"=w271:T10)
                n105 = call <vilib>:"Unflatten From JSON String.vi"("Type and Defaults"=w271, "error in (no error)"=w281, "JSON String"=w283) -> ("error out"=w284:errorcluster, "Variant"=w285:variant)  [unwired: 7 in]
                n106 = Variant To Data(error in=w284, type=w271, Variant=w285) -> (data=w282:T10, error out=w280:errorcluster)
                n107 = Unbundle By Name(w282) -> ("json.Method"=w273:string, "json.ArrayVar"=w275:string)
                n108 = property on="数组变量(ArrayVar)" class="Ring (strict)"() -> ("Strings []"=w276:string[])  [unwired: 2 in, 2 out]
                n109 = Search 1D Array(1D array=w276, element=w275) -> (index of element=w278:i32)  [unwired: 1 in]
                n110 = Greater Or Equal To 0?(x=w278) -> (x >= 0?=w277:bool)
                n111 = Select(t=w278, s=w277, f=0) -> (s? t:f=w274:i32)
                n112 = property on="数组变量(ArrayVar)" class="Ring (strict)"("Value"=w274) -> ()  [unwired: 2 in, 2 out]
              }
              frame "ArrayIndex" {
                n113 = Unbundle By Name(w287) -> ("IndexArray"=w286:T11)
                n114 = call <vilib>:"Unflatten From JSON String.vi"("Type and Defaults"=w286, "error in (no error)"=w297, "JSON String"=w299) -> ("error out"=w300:errorcluster, "Variant"=w301:variant)  [unwired: 7 in]
                n115 = Variant To Data(error in=w300, type=w286, Variant=w301) -> (data=w298:T11, error out=w296:errorcluster)
                n116 = Unbundle By Name(w298) -> ("json.Method"=w288:string, "json.ArrayVar"=w291:string, "json.Index"=w289:i32)
                n117 = local write "索引_ArrayIndex"(w289) -> ()
                n118 = property on="数组变量(ArrayVar)" class="Ring (strict)"() -> ("Strings []"=w292:string[])  [unwired: 2 in, 2 out]
                n119 = Search 1D Array(1D array=w292, element=w291) -> (index of element=w294:i32)  [unwired: 1 in]
                n120 = Greater Or Equal To 0?(x=w294) -> (x >= 0?=w293:bool)
                n121 = Select(t=w294, s=w293, f=0) -> (s? t:f=w290:i32)
                n122 = property on="数组变量(ArrayVar)" class="Ring (strict)"("Value"=w290) -> ()  [unwired: 2 in, 2 out]
              }
              frame "BuildArray" {
                n123 = Unbundle By Name(w306) -> ("BuildArray"=w305:T12)
                n124 = call <vilib>:"Unflatten From JSON String.vi"("Type and Defaults"=w305, "error in (no error)"=w309, "JSON String"=w311) -> ("error out"=w312:errorcluster, "Variant"=w313:variant)  [unwired: 7 in]
                n125 = Variant To Data(error in=w312, type=w305, Variant=w313) -> (data=w310:T12, error out=w308:errorcluster)
                n126 = Unbundle By Name(w310) -> ("json.Method"=w307:string, "json.FirstElementVar"=w303:string, "json.SecondElementVar"=w302:string)
                n127 = local write "第一个元素_BuildArray"(w303) -> ()
                n128 = local write "第二个元素_BuildArray"(w302) -> ()
                n129 = property on="数组变量(ArrayVar)" class="Ring (strict)"("Value"=0) -> ()  [unwired: 2 in, 2 out]
              }
              frame "InsertIntoArray" {
                n130 = Unbundle By Name(w323) -> ("InsertIntoArray"=w322:T13)
                n131 = call <vilib>:"Unflatten From JSON String.vi"("Type and Defaults"=w322, "error in (no error)"=w326, "JSON String"=w328) -> ("error out"=w329:errorcluster, "Variant"=w330:variant)  [unwired: 7 in]
                n132 = Variant To Data(error in=w329, type=w322, Variant=w330) -> (data=w327:T13, error out=w325:errorcluster)
                n133 = Unbundle By Name(w327) -> ("json.Method"=w324:string, "json.ArrayVar"=w316:string, "json.Index"=w315:i32, "json.SubArrayVar"=w314:string)
                n134 = property on="数组变量(ArrayVar)" class="Ring (strict)"() -> ("Strings []"=w319:string[])  [unwired: 2 in, 2 out]
                n135 = local write "尺寸_InitializeArray"(w315) -> ()
                n136 = local write "子数组_InsertIntoArray"(w314) -> ()
                n137 = Search 1D Array(1D array=w319, element=w316) -> (index of element=w321:i32)  [unwired: 1 in]
                n138 = Greater Or Equal To 0?(x=w321) -> (x >= 0?=w320:bool)
                n139 = Select(t=w321, s=w320, f=0) -> (s? t:f=w317:i32)
                n140 = property on="数组变量(ArrayVar)" class="Ring (strict)"("Value"=w317) -> ()  [unwired: 2 in, 2 out]
              }
              frame "DeleteFromArray" {
                n141 = Unbundle By Name(w340) -> ("DeleteFromArray"=w339:T14)
                n142 = call <vilib>:"Unflatten From JSON String.vi"("Type and Defaults"=w339, "error in (no error)"=w343, "JSON String"=w345) -> ("error out"=w346:errorcluster, "Variant"=w347:variant)  [unwired: 7 in]
                n143 = Variant To Data(error in=w346, type=w339, Variant=w347) -> (data=w344:T14, error out=w342:errorcluster)
                n144 = Unbundle By Name(w344) -> ("json.Method"=w341:string, "json.ArrayVar"=w333:string, "json.Index"=w332:i32, "json.Length"=w331:i32)
                n145 = local write "索引_DeleteFromArray"(w332) -> ()
                n146 = local write "删除长度_DeleteFromArray"(w331) -> ()
                n147 = property on="数组变量(ArrayVar)" class="Ring (strict)"() -> ("Strings []"=w336:string[])  [unwired: 2 in, 2 out]
                n148 = Search 1D Array(1D array=w336, element=w333) -> (index of element=w338:i32)  [unwired: 1 in]
                n149 = Greater Or Equal To 0?(x=w338) -> (x >= 0?=w337:bool)
                n150 = Select(t=w338, s=w337, f=0) -> (s? t:f=w334:i32)
                n151 = property on="数组变量(ArrayVar)" class="Ring (strict)"("Value"=w334) -> ()  [unwired: 2 in, 2 out]
              }
              frame "InitializeArray" {
                n152 = Unbundle By Name(w352) -> ("InitializeArray"=w351:T15)
                n153 = call <vilib>:"Unflatten From JSON String.vi"("Type and Defaults"=w351, "error in (no error)"=w355, "JSON String"=w357) -> ("error out"=w358:errorcluster, "Variant"=w359:variant)  [unwired: 7 in]
                n154 = Variant To Data(error in=w358, type=w351, Variant=w359) -> (data=w356:T15, error out=w354:errorcluster)
                n155 = Unbundle By Name(w356) -> ("json.Method"=w353:string, "json.ElementVar"=w348:string, "json.DimensionSize"=w349:i32)
                n156 = local write "尺寸_InitializeArray"(w349) -> ()
                n157 = property on="元素_InitializeArray" class="CmbBox"("Value"=w348) -> ()  [unwired: 2 in, 2 out]
                n158 = property on="数组变量(ArrayVar)" class="Ring (strict)"("Value"=0 ("f")) -> ()  [unwired: 2 in, 2 out]
              }
              frame "ArraySubset" {
                n159 = Unbundle By Name(w369) -> ("ArraySubset"=w368:T14)
                n160 = call <vilib>:"Unflatten From JSON String.vi"("Type and Defaults"=w368, "error in (no error)"=w372, "JSON String"=w374) -> ("error out"=w375:errorcluster, "Variant"=w376:variant)  [unwired: 7 in]
                n161 = Variant To Data(error in=w375, type=w368, Variant=w376) -> (data=w373:T14, error out=w371:errorcluster)
                n162 = Unbundle By Name(w373) -> ("json.Method"=w370:string, "json.ArrayVar"=w362:string, "json.Index"=w361:i32, "json.Length"=w360:i32)
                n163 = local write "索引_ArraySubset"(w361) -> ()
                n164 = local write "长度_ArraySubset"(w360) -> ()
                n165 = property on="数组变量(ArrayVar)" class="Ring (strict)"() -> ("Strings []"=w365:string[])  [unwired: 2 in, 2 out]
                n166 = Search 1D Array(1D array=w365, element=w362) -> (index of element=w367:i32)  [unwired: 1 in]
                n167 = Greater Or Equal To 0?(x=w367) -> (x >= 0?=w366:bool)
                n168 = Select(t=w367, s=w366, f=0) -> (s? t:f=w364:i32)
                n169 = property on="数组变量(ArrayVar)" class="Ring (strict)"("Value"=w364) -> ()  [unwired: 2 in, 2 out]
              }
              frame "ArrayMax" {
                n170 = Unbundle By Name(w384) -> ("ArrayMax"=w383:T10)
                n171 = call <vilib>:"Unflatten From JSON String.vi"("Type and Defaults"=w383, "error in (no error)"=w387, "JSON String"=w389) -> ("error out"=w390:errorcluster, "Variant"=w391:variant)  [unwired: 7 in]
                n172 = Variant To Data(error in=w390, type=w383, Variant=w391) -> (data=w388:T10, error out=w386:errorcluster)
                n173 = Unbundle By Name(w388) -> ("json.Method"=w385:string, "json.ArrayVar"=w377:string)
                n174 = property on="数组变量(ArrayVar)" class="Ring (strict)"() -> ("Strings []"=w380:string[])  [unwired: 2 in, 2 out]
                n175 = Search 1D Array(1D array=w380, element=w377) -> (index of element=w382:i32)  [unwired: 1 in]
                n176 = Greater Or Equal To 0?(x=w382) -> (x >= 0?=w381:bool)
                n177 = Select(t=w382, s=w381, f=0) -> (s? t:f=w379:i32)
                n178 = property on="数组变量(ArrayVar)" class="Ring (strict)"("Value"=w379) -> ()  [unwired: 2 in, 2 out]
              }
              frame "ArrayMin" {
                n179 = Unbundle By Name(w399) -> ("ArrayMax"=w398:T10)
                n180 = call <vilib>:"Unflatten From JSON String.vi"("Type and Defaults"=w398, "error in (no error)"=w402, "JSON String"=w404) -> ("error out"=w405:errorcluster, "Variant"=w406:variant)  [unwired: 7 in]
                n181 = Variant To Data(error in=w405, type=w398, Variant=w406) -> (data=w403:T10, error out=w401:errorcluster)
                n182 = Unbundle By Name(w403) -> ("json.Method"=w400:string, "json.ArrayVar"=w392:string)
                n183 = property on="数组变量(ArrayVar)" class="Ring (strict)"() -> ("Strings []"=w395:string[])  [unwired: 2 in, 2 out]
                n184 = Search 1D Array(1D array=w395, element=w392) -> (index of element=w397:i32)  [unwired: 1 in]
                n185 = Greater Or Equal To 0?(x=w397) -> (x >= 0?=w396:bool)
                n186 = Select(t=w397, s=w396, f=0) -> (s? t:f=w394:i32)
                n187 = property on="数组变量(ArrayVar)" class="Ring (strict)"("Value"=w394) -> ()  [unwired: 2 in, 2 out]
              }
              frame "SearchArray" {
                n188 = Unbundle By Name(w416) -> ("SearchArray"=w415:T16)
                n189 = call <vilib>:"Unflatten From JSON String.vi"("Type and Defaults"=w415, "error in (no error)"=w419, "JSON String"=w421) -> ("error out"=w422:errorcluster, "Variant"=w423:variant)  [unwired: 7 in]
                n190 = Variant To Data(error in=w422, type=w415, Variant=w423) -> (data=w420:T16, error out=w418:errorcluster)
                n191 = Unbundle By Name(w420) -> ("json.Method"=w417:string, "json.ArrayVar"=w409:string, "json.ElementVar"=w408:string, "json.StartIndex"=w407:i32)
                n192 = property on="数组变量(ArrayVar)" class="Ring (strict)"() -> ("Strings []"=w412:string[])  [unwired: 2 in, 2 out]
                n193 = local write "元素_SearchArray"(w408) -> ()
                n194 = local write "起始索引_SearchArray"(w407) -> ()
                n195 = Search 1D Array(1D array=w412, element=w409) -> (index of element=w414:i32)  [unwired: 1 in]
                n196 = Greater Or Equal To 0?(x=w414) -> (x >= 0?=w413:bool)
                n197 = Select(t=w414, s=w413, f=0) -> (s? t:f=w411:i32)
                n198 = property on="数组变量(ArrayVar)" class="Ring (strict)"("Value"=w411) -> ()  [unwired: 2 in, 2 out]
              }
              frame "ReplaceArraySubset" {
                n199 = Unbundle By Name(w433) -> ("ReplaceArraySubset"=w432:T13)
                n200 = call <vilib>:"Unflatten From JSON String.vi"("Type and Defaults"=w432, "error in (no error)"=w436, "JSON String"=w438) -> ("error out"=w439:errorcluster, "Variant"=w440:variant)  [unwired: 7 in]
                n201 = Variant To Data(error in=w439, type=w432, Variant=w440) -> (data=w437:T13, error out=w435:errorcluster)
                n202 = Unbundle By Name(w437) -> ("json.Method"=w434:string, "json.ArrayVar"=w426:string, "json.Index"=w425:i32, "json.SubArrayVar"=w424:string)
                n203 = local write "子数组_ReplaceArraySubset"(w424) -> ()
                n204 = property on="数组变量(ArrayVar)" class="Ring (strict)"() -> ("Strings []"=w429:string[])  [unwired: 2 in, 2 out]
                n205 = local write "索引_ReplaceArraySubset"(w425) -> ()
                n206 = Search 1D Array(1D array=w429, element=w426) -> (index of element=w431:i32)  [unwired: 1 in]
                n207 = Greater Or Equal To 0?(x=w431) -> (x >= 0?=w430:bool)
                n208 = Select(t=w431, s=w430, f=0) -> (s? t:f=w428:i32)
                n209 = property on="数组变量(ArrayVar)" class="Ring (strict)"("Value"=w428) -> ()  [unwired: 2 in, 2 out]
              }
              frame "SortArray" {
                n210 = Unbundle By Name(w448) -> ("SortArray"=w447:T10)
                n211 = call <vilib>:"Unflatten From JSON String.vi"("Type and Defaults"=w447, "error in (no error)"=w451, "JSON String"=w453) -> ("error out"=w454:errorcluster, "Variant"=w455:variant)  [unwired: 7 in]
                n212 = Variant To Data(error in=w454, type=w447, Variant=w455) -> (data=w452:T10, error out=w450:errorcluster)
                n213 = Unbundle By Name(w452) -> ("json.Method"=w449:string, "json.ArrayVar"=w441:string)
                n214 = property on="数组变量(ArrayVar)" class="Ring (strict)"() -> ("Strings []"=w444:string[])  [unwired: 2 in, 2 out]
                n215 = Search 1D Array(1D array=w444, element=w441) -> (index of element=w446:i32)  [unwired: 1 in]
                n216 = Greater Or Equal To 0?(x=w446) -> (x >= 0?=w445:bool)
                n217 = Select(t=w446, s=w445, f=0) -> (s? t:f=w443:i32)
                n218 = property on="数组变量(ArrayVar)" class="Ring (strict)"("Value"=w443) -> ()  [unwired: 2 in, 2 out]
              }
              frame "ReverseArray" {
                n219 = Unbundle By Name(w463) -> ("ReverseArray"=w462:T10)
                n220 = call <vilib>:"Unflatten From JSON String.vi"("Type and Defaults"=w462, "error in (no error)"=w466, "JSON String"=w468) -> ("error out"=w469:errorcluster, "Variant"=w470:variant)  [unwired: 7 in]
                n221 = Variant To Data(error in=w469, type=w462, Variant=w470) -> (data=w467:T10, error out=w465:errorcluster)
                n222 = Unbundle By Name(w467) -> ("json.Method"=w464:string, "json.ArrayVar"=w456:string)
                n223 = property on="数组变量(ArrayVar)" class="Ring (strict)"() -> ("Strings []"=w459:string[])  [unwired: 2 in, 2 out]
                n224 = Search 1D Array(1D array=w459, element=w456) -> (index of element=w461:i32)  [unwired: 1 in]
                n225 = Greater Or Equal To 0?(x=w461) -> (x >= 0?=w460:bool)
                n226 = Select(t=w461, s=w460, f=0) -> (s? t:f=w458:i32)
                n227 = property on="数组变量(ArrayVar)" class="Ring (strict)"("Value"=w458) -> ()  [unwired: 2 in, 2 out]
              }
              frame "ArrayAverage" {
                n228 = Unbundle By Name(w479) -> ("ArrayAverage"=w478:T17)
                n229 = call <vilib>:"Unflatten From JSON String.vi"("Type and Defaults"=w478, "error in (no error)"=w482, "JSON String"=w484) -> ("error out"=w485:errorcluster, "Variant"=w486:variant)  [unwired: 7 in]
                n230 = Variant To Data(error in=w485, type=w478, Variant=w486) -> (data=w483:T17, error out=w481:errorcluster)
                n231 = Unbundle By Name(w483) -> ("json.Method"=w480:string, "json.NumArrayVar"=w472:string, "json.IgnoreNaN"=w471:bool)
                n232 = local write "忽略NaN_ArrayAverage"(w471) -> ()
                n233 = property on="数组变量(ArrayVar)" class="Ring (strict)"() -> ("Strings []"=w475:string[])  [unwired: 2 in, 2 out]
                n234 = Search 1D Array(1D array=w475, element=w472) -> (index of element=w477:i32)  [unwired: 1 in]
                n235 = Greater Or Equal To 0?(x=w477) -> (x >= 0?=w476:bool)
                n236 = Select(t=w477, s=w476, f=0) -> (s? t:f=w474:i32)
                n237 = property on="数组变量(ArrayVar)" class="Ring (strict)"("Value"=w474) -> ()  [unwired: 2 in, 2 out]
              }
              frame "RemoveDuplicatesFromArray" {
                n238 = Unbundle By Name(w494) -> ("RemoveDuplicatesFromArray"=w493:T10)
                n239 = call <vilib>:"Unflatten From JSON String.vi"("Type and Defaults"=w493, "error in (no error)"=w497, "JSON String"=w499) -> ("error out"=w500:errorcluster, "Variant"=w501:variant)  [unwired: 7 in]
                n240 = Variant To Data(error in=w500, type=w493, Variant=w501) -> (data=w498:T10, error out=w496:errorcluster)
                n241 = Unbundle By Name(w498) -> ("json.Method"=w495:string, "json.ArrayVar"=w487:string)
                n242 = property on="数组变量(ArrayVar)" class="Ring (strict)"() -> ("Strings []"=w490:string[])  [unwired: 2 in, 2 out]
                n243 = Search 1D Array(1D array=w490, element=w487) -> (index of element=w492:i32)  [unwired: 1 in]
                n244 = Greater Or Equal To 0?(x=w492) -> (x >= 0?=w491:bool)
                n245 = Select(t=w492, s=w491, f=0) -> (s? t:f=w489:i32)
                n246 = property on="数组变量(ArrayVar)" class="Ring (strict)"("Value"=w489) -> ()  [unwired: 2 in, 2 out]
              }
              frame "ArrayToString" {
                n247 = Unbundle By Name(w510) -> ("ArrayToString"=w509:T18)
                n248 = call <vilib>:"Unflatten From JSON String.vi"("Type and Defaults"=w509, "error in (no error)"=w513, "JSON String"=w515) -> ("error out"=w516:errorcluster, "Variant"=w517:variant)  [unwired: 7 in]
                n249 = Variant To Data(error in=w516, type=w509, Variant=w517) -> (data=w514:T18, error out=w512:errorcluster)
                n250 = Unbundle By Name(w514) -> ("json.Method"=w511:string, "json.ArrayVar"=w503:string, "json.Delimiter"=w502:string)
                n251 = local write "分隔符_ArrayToString"(w502) -> ()
                n252 = property on="数组变量(ArrayVar)" class="Ring (strict)"() -> ("Strings []"=w506:string[])  [unwired: 2 in, 2 out]
                n253 = Search 1D Array(1D array=w506, element=w503) -> (index of element=w508:i32)  [unwired: 1 in]
                n254 = Greater Or Equal To 0?(x=w508) -> (x >= 0?=w507:bool)
                n255 = Select(t=w508, s=w507, f=0) -> (s? t:f=w505:i32)
                n256 = property on="数组变量(ArrayVar)" class="Ring (strict)"("Value"=w505) -> ()  [unwired: 2 in, 2 out]
              }
              frame Default {
              }
            }
            n257 = property on="方法(Method)" class="Enum (strict)"() -> ("Strings []"=w260:string[])  [unwired: 2 in, 2 out]
            n258 = Search 1D Array(1D array=w260, element=w258) -> (index of element=w262:i32)  [unwired: 1 in]
            n259 = Greater Or Equal To 0?(x=w262) -> (x >= 0?=w261:bool)
            n260 = Select(t=w262, s=w261, f=0) -> (s? t:f=w257:i32)
            n261 = local write "ArrayType"(w257) -> ()
            n262 = property on="方法(Method)" class="Enum (strict)"("Value"=w257) -> ()  [unwired: 2 in, 2 out]
          }
          frame True {
          }
        }
        n263 = call <vilib>:"Add State(s) to Queue__JKI_lib_State_Machine.vi"("State(s) in (\"\")"=w256) -> ("States Out"=w255:string)  [unwired: 14 in]
      }
      frame "Parameter: Combin Parameter" {
        n264 = property on="方法(Method)" class="Enum (strict)"() -> ("RingText.Text"=w521:string)  [unwired: 2 in, 2 out]
        n265 = case shown="\"ArrayToString\"" w521 {
          selector: w521 -> [_ w530 w539 w551 w562 w573 w583 w594 w603 w612 w623 w634 w643 w652 w662 w671 w681]
          tunnel: w524 -> [_ w537 w547 w557 w568 w579 w589 w600 w609 w618 w629 w640 w649 w658 w668 w677 w687]
          tunnel: [_ w535 w545 w555 w566 w577 w587 w598 w607 w616 w627 w638 w647 w656 w666 w675 w685] -> w520
          tunnel: [w528 w529 w538 w550 w561 w572 w582 w593 w602 w611 w622 w633 w642 w651 w661 w670 w680] -> w523
          tunnel: w522 -> [w528 w533 w543 w553 w564 w575 w585 w596 w605 w614 w625 w636 w645 w654 w664 w673 w683]
          frame Default {
          }
          frame "ArraySize" {
            n266 = property on="数组变量(ArrayVar)" class="Ring (strict)"() -> ("RingText.Text"=w532:string)  [unwired: 2 in, 2 out]
            n267 = Unbundle By Name(w537) -> ("ArrayClusters.ArraySize"=w536:T10)
            n268 = Bundle By Name(cluster=w536, "json.Method"=w530, "json.ArrayVar"=w532) -> (w531:T10)
            n269 = call <vilib>:"Flatten To JSON String.vi"("Multiline (T)"=TRUE, "error in (no error)"=w533, "Variant"=w531) -> ("error out"=w529:errorcluster, "JSON String"=w535:string)  [unwired: 7 in]
          }
          frame "ArrayIndex" {
            n270 = property on="数组变量(ArrayVar)" class="Ring (strict)"() -> ("RingText.Text"=w542:string)  [unwired: 2 in, 2 out]
            n271 = Unbundle By Name(w547) -> ("ArrayClusters.IndexArray"=w546:T11)
            n272 = local read "索引_ArrayIndex"() -> (w541:u32)
            n273 = Bundle By Name(cluster=w546, "json.Method"=w539, "json.ArrayVar"=w542, "json.Index"=w541) -> (w540:T11)
            n274 = call <vilib>:"Flatten To JSON String.vi"("Multiline (T)"=TRUE, "error in (no error)"=w543, "Variant"=w540) -> ("error out"=w538:errorcluster, "JSON String"=w545:string)  [unwired: 7 in]
          }
          frame "BuildArray" {
            n275 = local read "第二个元素_BuildArray"() -> (w548:string)
            n276 = local read "第一个元素_BuildArray"() -> (w549:string)
            n277 = Unbundle By Name(w557) -> ("ArrayClusters.BuildArray"=w556:T12)
            n278 = Bundle By Name(cluster=w556, "json.Method"=w551, "json.FirstElementVar"=w549, "json.SecondElementVar"=w548) -> (w552:T12)
            n279 = call <vilib>:"Flatten To JSON String.vi"("Multiline (T)"=TRUE, "error in (no error)"=w553, "Variant"=w552) -> ("error out"=w550:errorcluster, "JSON String"=w555:string)  [unwired: 7 in]
          }
          frame "InsertIntoArray" {
            n280 = local read "子数组_InsertIntoArray"() -> (w558:string)
            n281 = local read "索引_InsertIntoArray"() -> (w559:u32)
            n282 = property on="数组变量(ArrayVar)" class="Ring (strict)"() -> ("RingText.Text"=w560:string)  [unwired: 2 in, 2 out]
            n283 = Unbundle By Name(w568) -> ("ArrayClusters.InsertIntoArray"=w567:T13)
            n284 = Bundle By Name(cluster=w567, "json.Method"=w562, "json.ArrayVar"=w560, "json.Index"=w559, "json.SubArrayVar"=w558) -> (w563:T13)
            n285 = call <vilib>:"Flatten To JSON String.vi"("Multiline (T)"=TRUE, "error in (no error)"=w564, "Variant"=w563) -> ("error out"=w561:errorcluster, "JSON String"=w566:string)  [unwired: 7 in]
          }
          frame "DeleteFromArray" {
            n286 = local read "删除长度_DeleteFromArray"() -> (w569:u32)
            n287 = property on="数组变量(ArrayVar)" class="Ring (strict)"() -> ("RingText.Text"=w571:string)  [unwired: 2 in, 2 out]
            n288 = local read "索引_DeleteFromArray"() -> (w570:u32)
            n289 = Unbundle By Name(w579) -> ("ArrayClusters.DeleteFromArray"=w578:T14)
            n290 = Bundle By Name(cluster=w578, "json.Method"=w573, "json.ArrayVar"=w571, "json.Index"=w570, "json.Length"=w569) -> (w574:T14)
            n291 = call <vilib>:"Flatten To JSON String.vi"("Multiline (T)"=TRUE, "error in (no error)"=w575, "Variant"=w574) -> ("error out"=w572:errorcluster, "JSON String"=w577:string)  [unwired: 7 in]
          }
          frame "InitializeArray" {
            n292 = local read "元素_InitializeArray"() -> (w581:string)
            n293 = local read "尺寸_InitializeArray"() -> (w580:u32)
            n294 = Unbundle By Name(w589) -> ("ArrayClusters.InitializeArray"=w588:T15)
            n295 = Bundle By Name(cluster=w588, "json.Method"=w583, "json.ElementVar"=w581, "json.DimensionSize"=w580) -> (w584:T15)
            n296 = call <vilib>:"Flatten To JSON String.vi"("Multiline (T)"=TRUE, "error in (no error)"=w585, "Variant"=w584) -> ("error out"=w582:errorcluster, "JSON String"=w587:string)  [unwired: 7 in]
          }
          frame "ArraySubset" {
            n297 = local read "长度_ArraySubset"() -> (w590:u32)
            n298 = local read "索引_ArraySubset"() -> (w591:u32)
            n299 = property on="数组变量(ArrayVar)" class="Ring (strict)"() -> ("RingText.Text"=w592:string)  [unwired: 2 in, 2 out]
            n300 = Unbundle By Name(w600) -> ("ArrayClusters.ArraySubset"=w599:T14)
            n301 = Bundle By Name(cluster=w599, "json.Method"=w594, "json.ArrayVar"=w592, "json.Index"=w591, "json.Length"=w590) -> (w595:T14)
            n302 = call <vilib>:"Flatten To JSON String.vi"("Multiline (T)"=TRUE, "error in (no error)"=w596, "Variant"=w595) -> ("error out"=w593:errorcluster, "JSON String"=w598:string)  [unwired: 7 in]
          }
          frame "ArrayMax" {
            n303 = property on="数组变量(ArrayVar)" class="Ring (strict)"() -> ("RingText.Text"=w601:string)  [unwired: 2 in, 2 out]
            n304 = Unbundle By Name(w609) -> ("ArrayClusters.ArrayMax"=w608:T10)
            n305 = Bundle By Name(cluster=w608, "json.Method"=w603, "json.ArrayVar"=w601) -> (w604:T10)
            n306 = call <vilib>:"Flatten To JSON String.vi"("Multiline (T)"=TRUE, "error in (no error)"=w605, "Variant"=w604) -> ("error out"=w602:errorcluster, "JSON String"=w607:string)  [unwired: 7 in]
          }
          frame "ArrayMin" {
            n307 = property on="数组变量(ArrayVar)" class="Ring (strict)"() -> ("RingText.Text"=w610:string)  [unwired: 2 in, 2 out]
            n308 = Unbundle By Name(w618) -> ("ArrayClusters.ArrayMin"=w617:T10)
            n309 = Bundle By Name(cluster=w617, "json.Method"=w612, "json.ArrayVar"=w610) -> (w613:T10)
            n310 = call <vilib>:"Flatten To JSON String.vi"("Multiline (T)"=TRUE, "error in (no error)"=w614, "Variant"=w613) -> ("error out"=w611:errorcluster, "JSON String"=w616:string)  [unwired: 7 in]
          }
          frame "SearchArray" {
            n311 = local read "起始索引_SearchArray"() -> (w619:u32)
            n312 = local read "元素_SearchArray"() -> (w620:string)
            n313 = property on="数组变量(ArrayVar)" class="Ring (strict)"() -> ("RingText.Text"=w621:string)  [unwired: 2 in, 2 out]
            n314 = Unbundle By Name(w629) -> ("ArrayClusters.SearchArray"=w628:T16)
            n315 = Bundle By Name(cluster=w628, "json.Method"=w623, "json.ArrayVar"=w621, "json.ElementVar"=w620, "json.StartIndex"=w619) -> (w624:T16)
            n316 = call <vilib>:"Flatten To JSON String.vi"("Multiline (T)"=TRUE, "error in (no error)"=w625, "Variant"=w624) -> ("error out"=w622:errorcluster, "JSON String"=w627:string)  [unwired: 7 in]
          }
          frame "ReplaceArraySubset" {
            n317 = local read "子数组_ReplaceArraySubset"() -> (w630:string)
            n318 = local read "索引_ReplaceArraySubset"() -> (w631:u32)
            n319 = property on="数组变量(ArrayVar)" class="Ring (strict)"() -> ("RingText.Text"=w632:string)  [unwired: 2 in, 2 out]
            n320 = Unbundle By Name(w640) -> ("ArrayClusters.ReplaceArraySubset"=w639:T13)
            n321 = Bundle By Name(cluster=w639, "json.Method"=w634, "json.ArrayVar"=w632, "json.Index"=w631, "json.SubArrayVar"=w630) -> (w635:T13)
            n322 = call <vilib>:"Flatten To JSON String.vi"("Multiline (T)"=TRUE, "error in (no error)"=w636, "Variant"=w635) -> ("error out"=w633:errorcluster, "JSON String"=w638:string)  [unwired: 7 in]
          }
          frame "SortArray" {
            n323 = property on="数组变量(ArrayVar)" class="Ring (strict)"() -> ("RingText.Text"=w641:string)  [unwired: 2 in, 2 out]
            n324 = Unbundle By Name(w649) -> ("ArrayClusters.SortArray"=w648:T10)
            n325 = Bundle By Name(cluster=w648, "json.Method"=w643, "json.ArrayVar"=w641) -> (w644:T10)
            n326 = call <vilib>:"Flatten To JSON String.vi"("Multiline (T)"=TRUE, "error in (no error)"=w645, "Variant"=w644) -> ("error out"=w642:errorcluster, "JSON String"=w647:string)  [unwired: 7 in]
          }
          frame "ReverseArray" {
            n327 = property on="数组变量(ArrayVar)" class="Ring (strict)"() -> ("RingText.Text"=w650:string)  [unwired: 2 in, 2 out]
            n328 = Unbundle By Name(w658) -> ("ArrayClusters.ReverseArray"=w657:T10)
            n329 = Bundle By Name(cluster=w657, "json.Method"=w652, "json.ArrayVar"=w650) -> (w653:T10)
            n330 = call <vilib>:"Flatten To JSON String.vi"("Multiline (T)"=TRUE, "error in (no error)"=w654, "Variant"=w653) -> ("error out"=w651:errorcluster, "JSON String"=w656:string)  [unwired: 7 in]
          }
          frame "ArrayAverage" {
            n331 = local read "忽略NaN_ArrayAverage"() -> (w659:bool)
            n332 = property on="数组变量(ArrayVar)" class="Ring (strict)"() -> ("RingText.Text"=w660:string)  [unwired: 2 in, 2 out]
            n333 = Unbundle By Name(w668) -> ("ArrayClusters.ArrayAverage"=w667:T17)
            n334 = Bundle By Name(cluster=w667, "json.Method"=w662, "json.NumArrayVar"=w660, "json.IgnoreNaN"=w659) -> (w663:T17)
            n335 = call <vilib>:"Flatten To JSON String.vi"("Multiline (T)"=TRUE, "error in (no error)"=w664, "Variant"=w663) -> ("error out"=w661:errorcluster, "JSON String"=w666:string)  [unwired: 7 in]
          }
          frame "RemoveDuplicatesFromArray" {
            n336 = property on="数组变量(ArrayVar)" class="Ring (strict)"() -> ("RingText.Text"=w669:string)  [unwired: 2 in, 2 out]
            n337 = Unbundle By Name(w677) -> ("ArrayClusters.RemoveDuplicatesFromArray"=w676:T10)
            n338 = Bundle By Name(cluster=w676, "json.Method"=w671, "json.ArrayVar"=w669) -> (w672:T10)
            n339 = call <vilib>:"Flatten To JSON String.vi"("Multiline (T)"=TRUE, "error in (no error)"=w673, "Variant"=w672) -> ("error out"=w670:errorcluster, "JSON String"=w675:string)  [unwired: 7 in]
          }
          frame "ArrayToString" {
            n340 = local read "分隔符_ArrayToString"() -> (w678:string)
            n341 = property on="数组变量(ArrayVar)" class="Ring (strict)"() -> ("RingText.Text"=w679:string)  [unwired: 2 in, 2 out]
            n342 = Unbundle By Name(w687) -> ("ArrayClusters.ArrayToString"=w686:T18)
            n343 = Bundle By Name(cluster=w686, "json.Method"=w681, "json.ArrayVar"=w679, "json.Delimiter"=w678) -> (w682:T18)
            n344 = call <vilib>:"Flatten To JSON String.vi"("Multiline (T)"=TRUE, "error in (no error)"=w683, "Variant"=w682) -> ("error out"=w680:errorcluster, "JSON String"=w685:string)  [unwired: 7 in]
          }
        }
        n345 = Bundle By Name(cluster=w524, "Synchronize.Echo.JsonOut"=w520) -> (w525:T7)
        n346 = call <vilib>:"Add State(s) to Queue__JKI_lib_State_Machine.vi"("State(s) in (\"\")"=w527) -> ("States Out"=w526:string)  [unwired: 14 in]
      }
      frame "---------- Sync ----------" {
        n347 = call <vilib>:"Add State(s) to Queue__JKI_lib_State_Machine.vi"("State(s) in (\"\")"=w691) -> ("States Out"=w690:string)  [unwired: 14 in]
      }
      frame "Sync: Obtain CMD Queue" {
        # "这里由平台输入"
        n348 = Unbundle By Name(w693) -> ("Synchronize.EnqueueData"=w692:T19)
        n349 = Obtain Queue(name (unnamed)="VIId", element data type=w692, error in (no error)=w698) -> (queue out=w694:refnum<queue>, error out=w697:errorcluster)  [unwired: 2 in, 1 out]
        n350 = Bundle By Name(cluster=w693, "Synchronize.Queue"=w694) -> (w695:T7)
        n351 = call <vilib>:"Add State(s) to Queue__JKI_lib_State_Machine.vi"("State(s) in (\"\")"=w700) -> ("States Out"=w699:string)  [unwired: 14 in]
      }
      frame "Sync: Dequeue CMD" {
        n352 = Unbundle By Name(w713) -> ("Synchronize.Queue"=w710:refnum<queue>, "Synchronize.Communicate"=w701:T20)
        n353 = Dequeue Element(queue=w710, timeout in ms (-1)=10, error in (no error)=w711) -> (queue out=w709:refnum<queue>, element=w707:T19, timed out?=w708:bool, error out=w703:errorcluster)
        n354 = Bundle By Name(cluster=w713, "Synchronize.Queue"=w709, "Synchronize.EnqueueData"=w707) -> (w705:T7)
        n355 = case shown="False" w708 {
          tunnel: w707 -> [w724 _]
          tunnel: [w722 _] -> w706
          tunnel: w705 -> [w721 w753]
          tunnel: [w720 w753] -> w704
          tunnel: w703 -> [w718 w752]
          tunnel: [w717 w752] -> w702
          tunnel: w701 -> [w716 _]
          frame False {
            n356 = Unbundle By Name(w724) -> ("Action"=w723:T21, "Data"=w719:variant)
            n357 = case shown="\"Query\"" w723 {
              tunnel: ["Sync: Send ECHO" "UI: Initialize VarList\nSync: Send ECHO" _ "Sync: Send ECHO\nMacro: Exit" "Parameter: Combin Parameter\nSync: Send ECHO" "Parameter: Parse Parameter\nSync: Send ECHO"] -> w722
              tunnel: w721 -> [w727 w732 w736 w739 w744 w749]
              tunnel: [w726 w731 w736 w738 w743 w748] -> w720
              tunnel: w719 -> [_ _ _ _ _ _]
              tunnel: w718 -> [w728 w733 w735 w740 w745 w750]
              tunnel: [w728 w733 w735 w740 w745 w750] -> w717
              tunnel: w716 -> [_ _ _ _ _ _]
              frame "Create" {
                n358 = Bundle By Name(cluster=w727, "Synchronize.Echo.Status"="Create Success") -> (w726:T7)
              }
              frame "UpdateVariable" {
                n359 = Bundle By Name(cluster=w732, "Synchronize.Echo.Status"="UpdateVariable Success") -> (w731:T7)
              }
              frame Default {
              }
              frame "Close" {
                n360 = Bundle By Name(cluster=w739, "Synchronize.Echo.Status"="Close Success") -> (w738:T7)
              }
              frame "Query" {
                n361 = Bundle By Name(cluster=w744, "Synchronize.Echo.Status"="Query Success") -> (w743:T7)
              }
              frame "Revert" {
                n362 = Bundle By Name(cluster=w749, "Synchronize.Echo.Status"="Revert Success") -> (w748:T7)
              }
            }
          }
          frame True {
          }
        }
        n363 = call <vilib>:"Add State(s) to Queue__JKI_lib_State_Machine.vi"("State(s) in Front (\"\")"=w706, "State(s) in (\"\")"=w715) -> ("States Out"=w714:string)  [unwired: 13 in]
      }
      frame "Sync: Release CMD Queue" {
        n364 = Unbundle By Name(w756) -> ("Synchronize.Queue"=w757:refnum<queue>)
        n365 = Release Queue(queue=w757, error in (no error)=w755) -> (error out=w754:errorcluster)  [unwired: 1 in, 2 out]
        n366 = call <vilib>:"Add State(s) to Queue__JKI_lib_State_Machine.vi"("State(s) in (\"\")"=w759) -> ("States Out"=w758:string)  [unwired: 14 in]
      }
      frame "Sync: Send ECHO" {
        n367 = Unbundle By Name(w763) -> ("Synchronize.Communicate"=w760:T20, "Synchronize.EnqueueData.Data"=w772:variant, "Synchronize.Echo"=w764:T22)
        n368 = Variant To Data(error in=w762, type=w760, Variant=w772) -> (data=w765:T20, error out=w766:errorcluster)
        n369 = Unbundle By Name(w765) -> ("ID"=w769:string)
        n370 = Obtain Queue(name (unnamed)=w769, element data type=w764, error in (no error)=w766) -> (queue out=w768:refnum<queue>, error out=w770:errorcluster)  [unwired: 2 in, 1 out]
        n371 = Enqueue Element(queue=w768, element=w764, error in (no error)=w770) -> (queue out=w767:refnum<queue>, error out=w771:errorcluster)  [unwired: 1 in, 1 out]
        n372 = Release Queue(queue=w767, error in (no error)=w771) -> (error out=w761:errorcluster)  [unwired: 1 in, 2 out]
        n373 = call <vilib>:"Add State(s) to Queue__JKI_lib_State_Machine.vi"("State(s) in (\"\")"=w774) -> ("States Out"=w773:string)  [unwired: 14 in]
      }
    }
  }
  n374 = flat-sequence {
    frame #0 {
    }
  }
